vi "Master_IMUMain.vi"(8 "error in":errorcluster, 11 "VISA Refnum out":refnum<visa-resource-name>) -> (0 "error out":errorcluster)   [LabVIEW 2018]
doc: "VI dedicated to reading and processing incoming data from IMU (SBG Ellipse)."
uses:
  TypeDef_LoopPeriods.ctl
  TypeDef_IMUData.ctl
panel:
  out "Data skipped":bool
  out "buffer length":i32
  out "msg_id":string
  # "."
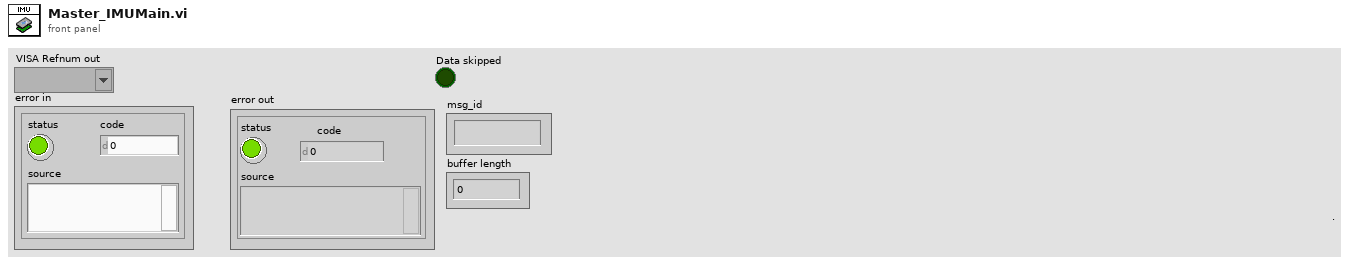
[diagram p1: front panel]
types:
  T1 = typedef "TypeDef_LoopPeriods.ctl" = cluster{"Control Period":i64, "DAQ Period":u32, "IMU Period":u32, "CAN Period":i64, "Nav Period":u32}
  T2 = typedef "TypeDef_IMUData.ctl" = cluster{"x acceleration (g)":dbl, "Pressure (psia)":dbl, "Temperature (F)":dbl}
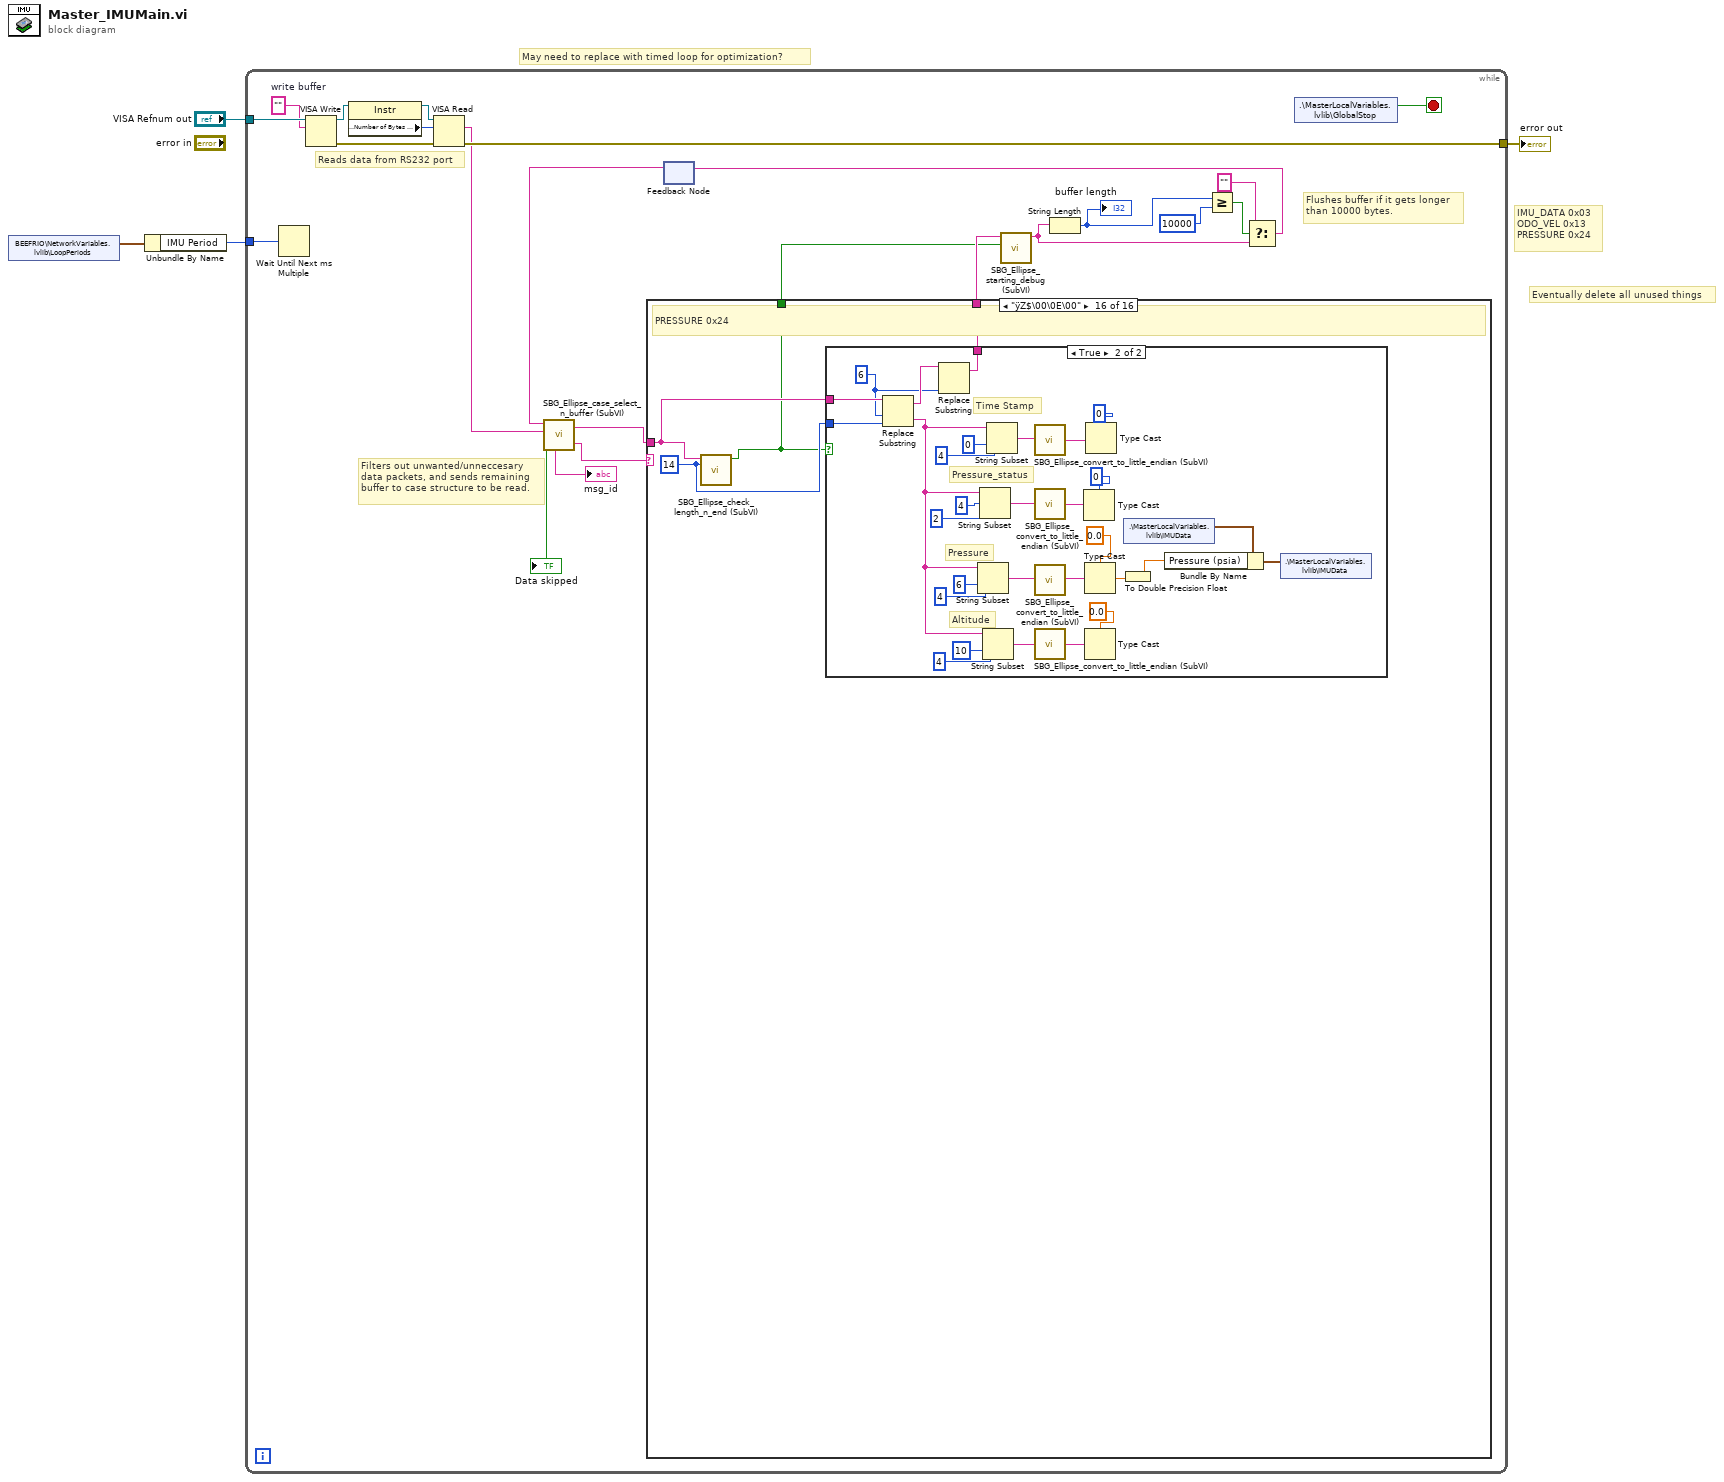
[diagram p0: block diagram]
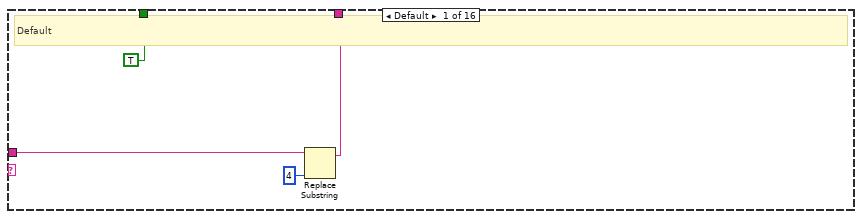
[diagram p2: hidden frame]
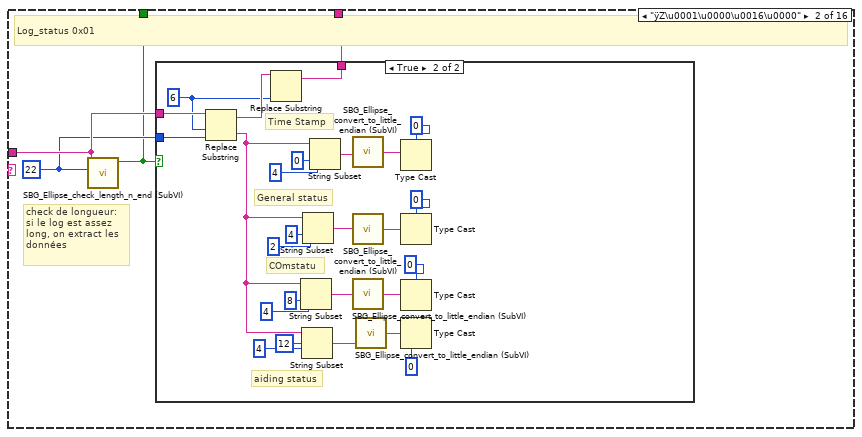
[diagram p3: hidden frame]
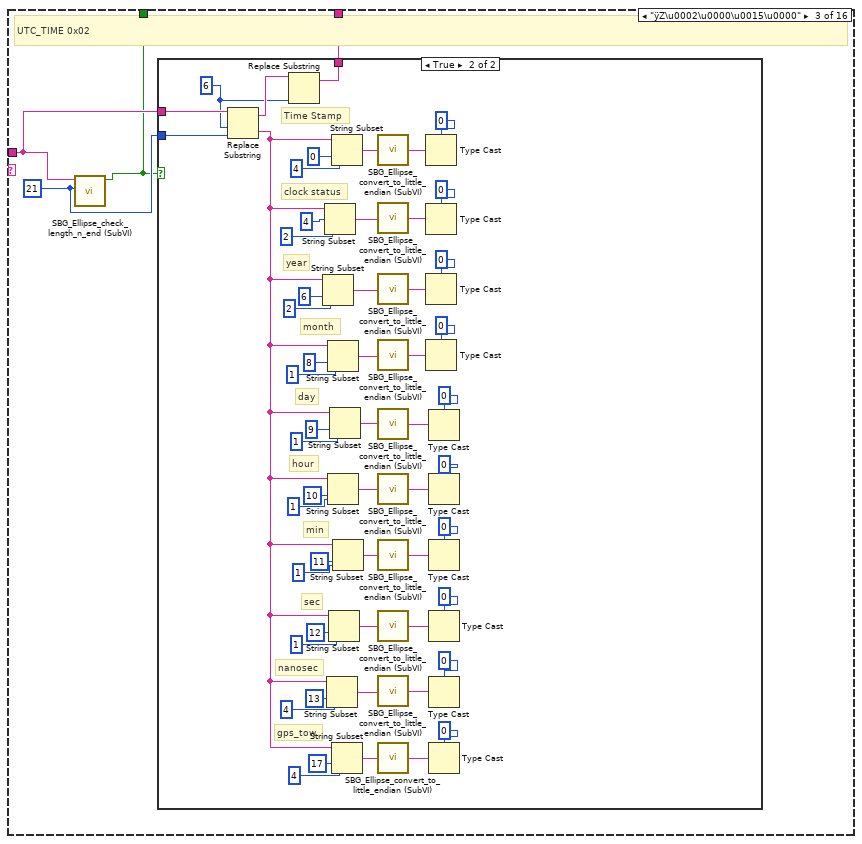
[diagram p5: hidden frame]
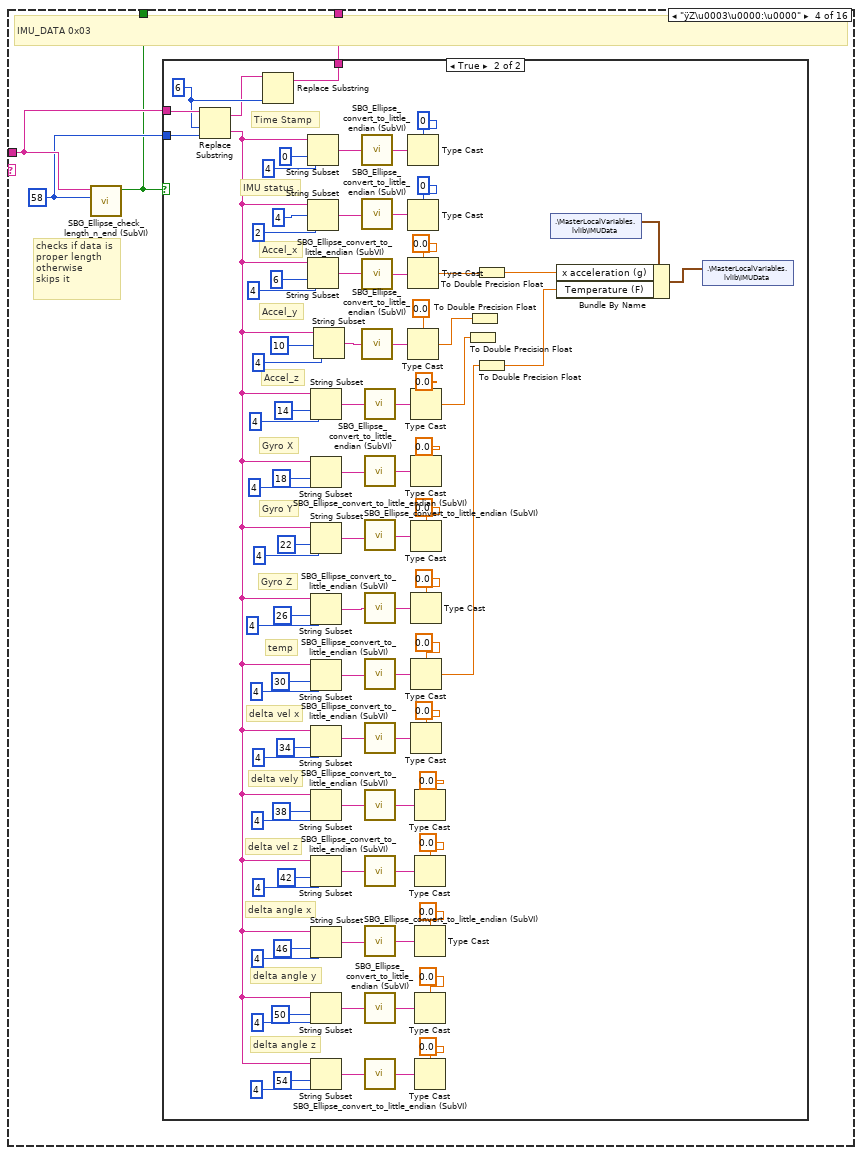
[diagram p7: hidden frame]
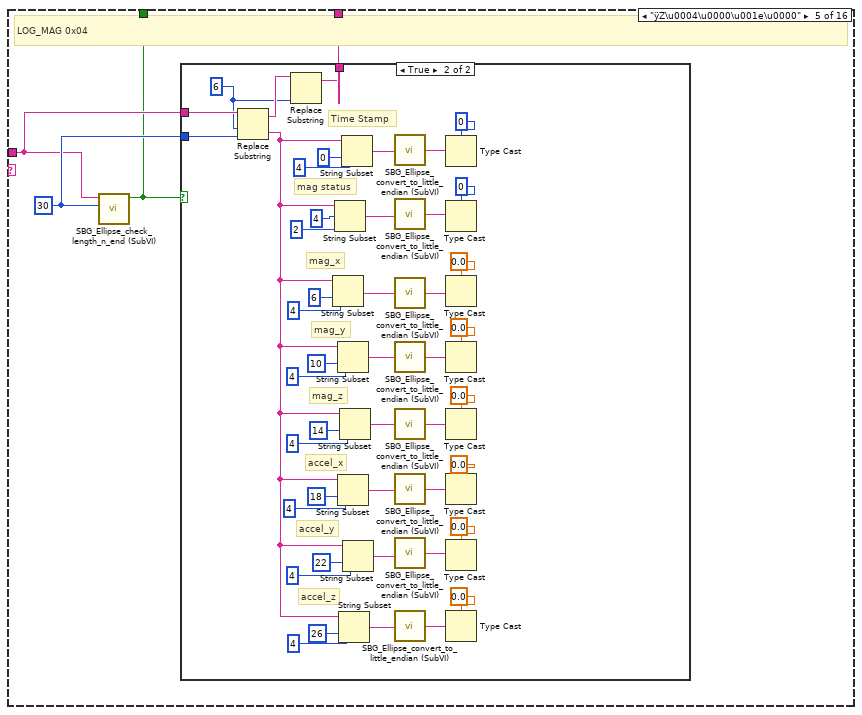
[diagram p9: hidden frame]
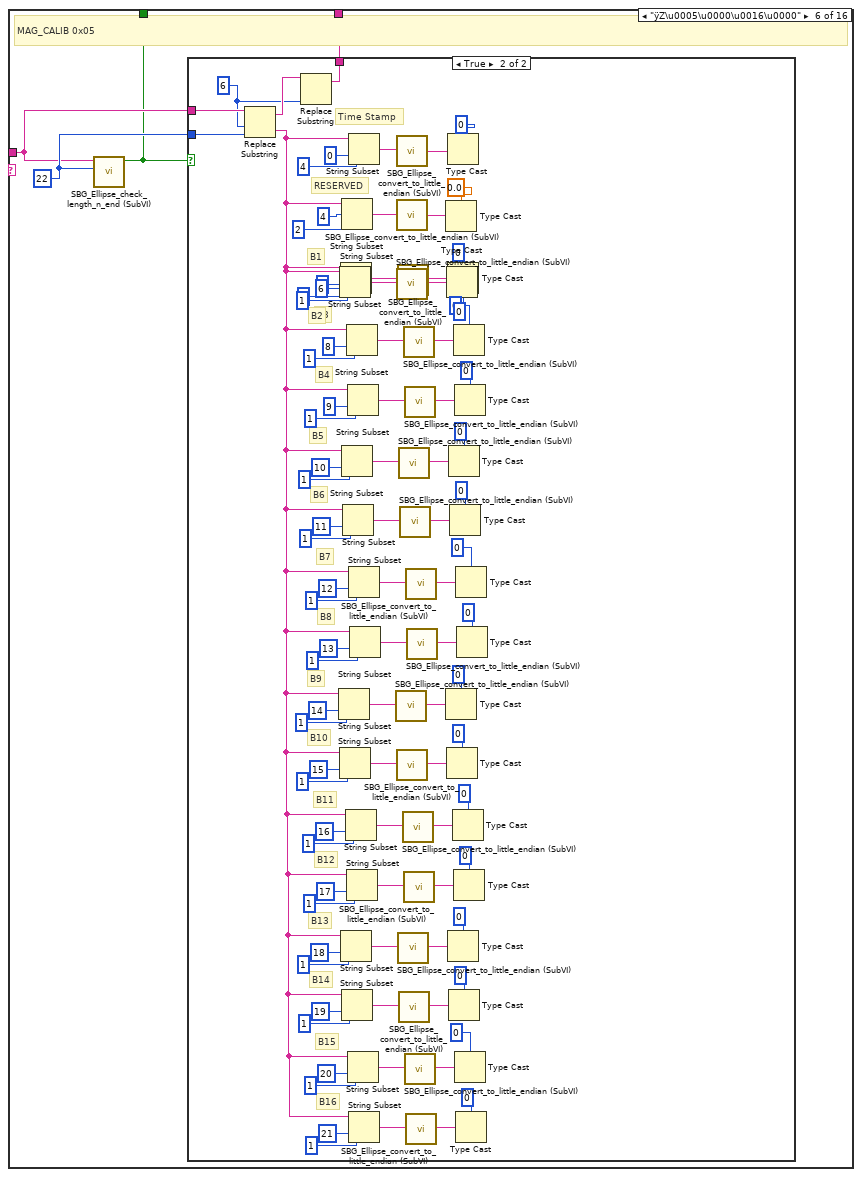
[diagram p11: hidden frame]
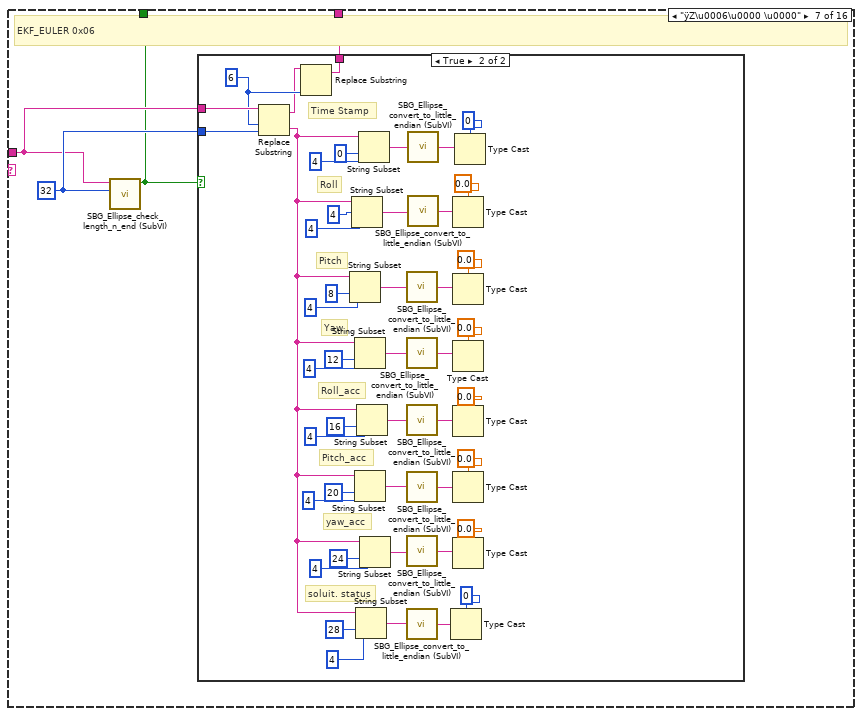
[diagram p13: hidden frame]
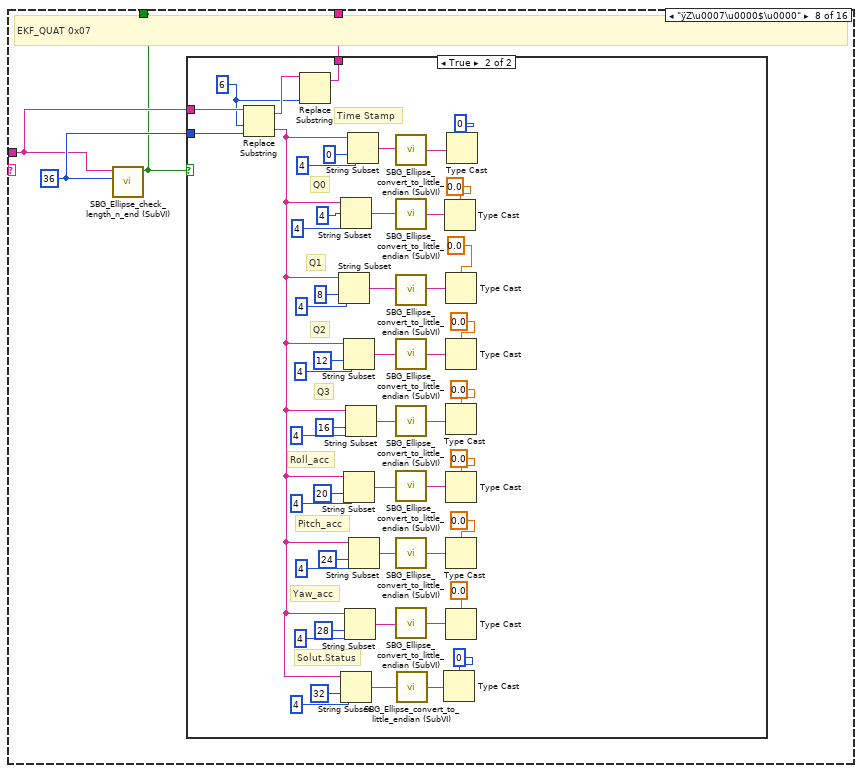
[diagram p15: hidden frame]
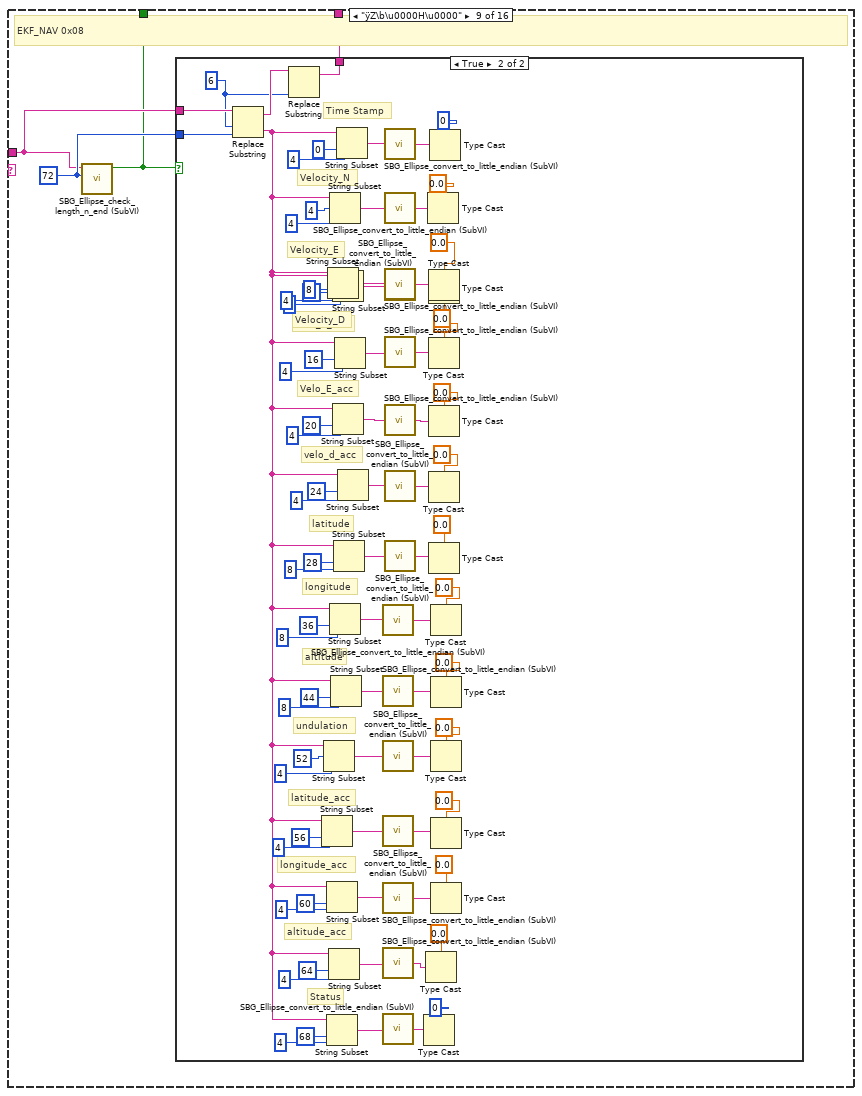
[diagram p17: hidden frame]
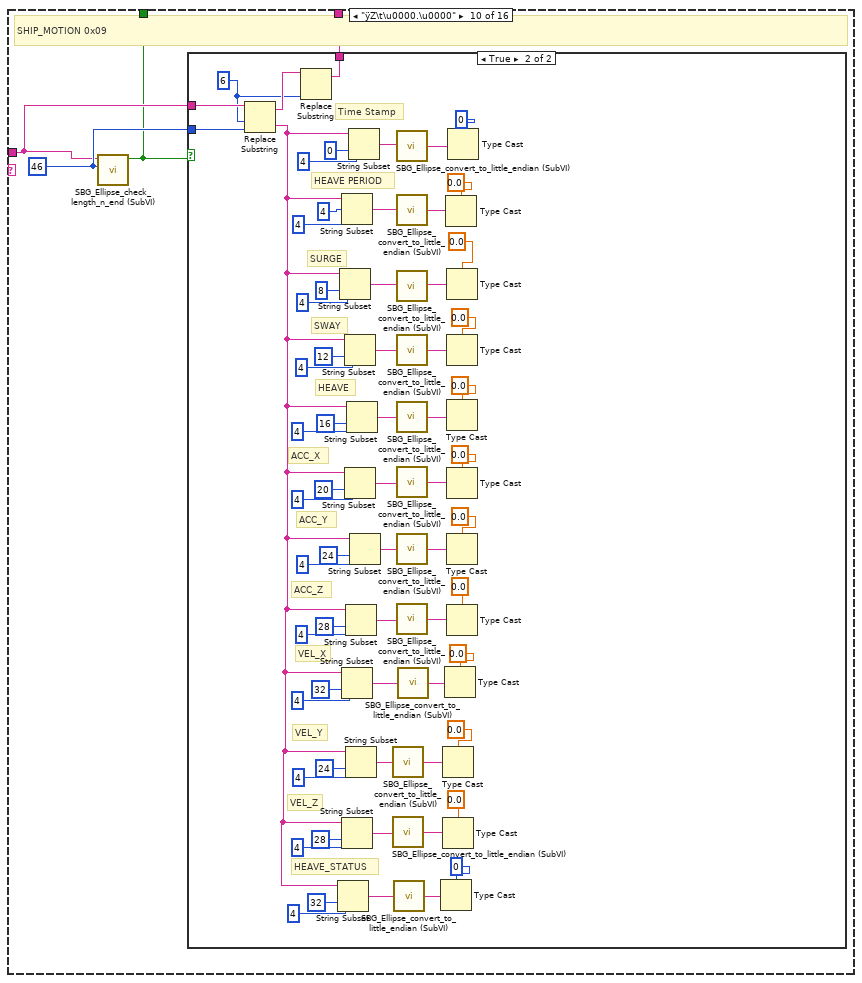
[diagram p19: hidden frame]
diagram:
  # "Eventually delete all unused things"
  # "May need to replace with timed loop for optimization?"
  # "IMU_DATA 0x03\nODO_VEL 0x13\nPRESSURE 0x24"
  n1 = shared-variable "BEEFRIO\\NetworkVariables.lvlib\\LoopPeriods"() -> (w2:T1)  [unwired: 1 in, 1 out]
  n2 = Unbundle By Name(w2) -> ("IMU Period"=w1:u32)
  n3 = while {
    tunnel: "VISA Refnum out" -> [w27]
    tunnel: [w21] -> w3
    tunnel: w1 -> [w11]
    stop <- w10 stop-if-true
    w22 = ""  # write buffer
    # "Filters out unwanted/unneccesary \ndata packets, and sends remaining\nbuffer to case structure to be read."
    # "Reads data from RS232 port"
    # "Flushes buffer if it gets longer\nthan 10000 bytes."
    n4 = Wait Until Next ms Multiple(millisecond multiple=w11) -> ()  [unwired: 1 out]
    n5 = VISA Write(VISA resource name=w27, write buffer=w22) -> (VISA resource name out=w23:refnum<visa-resource-name>, error out=w26:errorcluster)  [unwired: 1 in, 1 out]
    n6 = property class="Instr"(reference=w23) -> (reference out=w24:refnum<visa-resource-name>, "Serial Settings:Number of Bytes at Serial Port"=w25:u32)  [unwired: 1 in, 1 out]
    n7 = VISA Read(VISA resource name=w24, byte count=w25, error in (no error)=w26) -> (read buffer=w19:string, error out=w21:errorcluster)  [unwired: 2 out]
    n8 = feedback #1() -> (w20:string)  [unwired: 1 in]
    n9 = call "SBG_Ellipse_case_select_n_buffer (SubVI).vi"("new data in"=w19, "buffer data in"=w20) -> ("case_selector"=w7:string, "data out"=w8:string, "msg_id"=→"msg_id":string, "Data skipped"=→"Data skipped":bool)  [unwired: 2 in]
    n10 = case shown="\"ÿZ$\\00\\0E\\00\"" w7 {
      tunnel: w8 -> [w30 w34 w66 w126 w220 w271 w371 w423 w479 w565 w634 w702 w778 w824 w851 w892]
      tunnel: [w29 w35 w64 w127 w219 w270 w372 w422 w478 w563 w636 w701 w777 w823 w850 w891] -> w9
      tunnel: [TRUE ("Boolean") w32 w63 w124 w218 w269 w370 w421 w477 w564 w635 w700 w776 w822 w849 w890] -> w6
      frame Default {
        # "Default"
        n11 = Replace Substring(2:4 ("length (len. of substring)"), 5:w30) -> (1:w29:string)  [unwired: 2 in, 1 out]
      }
      frame "ÿZ\u0001\u0000\u0016\u0000" {
        w33 = 22 ("x")
        # "check de longueur:\nsi le log est assez\nlong, on extract les \ndonnées"
        # "Log_status 0x01"
        n12 = call "SBG_Ellipse_check_length_n_end (SubVI).vi"("x"=w33, "input String"=w34) -> ("is data ok?"=w32:bool)  [unwired: 7 in, 2 out]
        n13 = case shown="True" w32 {
          tunnel: w34 -> [w36 w62]
          tunnel: [w36 w45] -> w35
          tunnel: w33 -> [_ w52]
          frame False {
          }
          frame True {
            w46 = 6 ("length (len. of substring)")
            # "aiding status"
            # "COmstatu"
            # "General status"
            # "Time Stamp"
            n14 = Replace Substring(2:w52, 3:w46, 5:w62) -> (0:w61:string, 1:w47:string)  [unwired: 1 in]
            n15 = Replace Substring(2:w46, 5:w47) -> (1:w45:string)  [unwired: 2 in, 1 out]
            n16 = String Subset(string=w61, offset (0)=8 ("length (len. of substring)"), length (rest)=4 ("length (len. of substring)")) -> (substring=w43:string)
            n17 = String Subset(string=w61, offset (0)=12 ("length (len. of substring)"), length (rest)=4 ("length (len. of substring)")) -> (substring=w44:string)
            n18 = String Subset(string=w61, offset (0)=4 ("length (len. of substring)"), length (rest)=2 ("length (len. of substring)")) -> (substring=w42:string)
            n19 = String Subset(string=w61, offset (0)=0 ("length (len. of substring)"), length (rest)=4 ("length (len. of substring)")) -> (substring=w41:string)
            n20 = call "SBG_Ellipse_convert_to_little_endian (SubVI).vi"("string"=w41) -> ("String"=w40:string)  [unwired: 4 in]
            n21 = call "SBG_Ellipse_convert_to_little_endian (SubVI).vi"("string"=w42) -> ("String"=w39:string)  [unwired: 4 in]
            n22 = call "SBG_Ellipse_convert_to_little_endian (SubVI).vi"("string"=w43) -> ("String"=w38:string)  [unwired: 4 in]
            n23 = call "SBG_Ellipse_convert_to_little_endian (SubVI).vi"("string"=w44) -> ("String"=w37:string)  [unwired: 4 in]
            n24 = Type Cast(type=u32 0, x=w40) -> ()  [unwired: 1 out]
            n25 = Type Cast(type=u16 0, x=w39) -> ()  [unwired: 1 out]
            n26 = Type Cast(type=u32 0, x=w38) -> ()  [unwired: 1 out]
            n27 = Type Cast(type=u32 0, x=w37) -> ()  [unwired: 1 out]
          }
        }
      }
      frame "ÿZ\u0002\u0000\u0015\u0000" {
        w65 = 21 ("x")
        # "UTC_TIME 0x02"
        n28 = call "SBG_Ellipse_check_length_n_end (SubVI).vi"("x"=w65, "input String"=w66) -> ("is data ok?"=w63:bool)  [unwired: 7 in, 2 out]
        n29 = case shown="True" w63 {
          tunnel: w66 -> [w67 w123]
          tunnel: [w67 w88] -> w64
          tunnel: w65 -> [_ w101]
          frame False {
          }
          frame True {
            w89 = 6 ("length (len. of substring)")
            # "gps_tow"
            # "nanosec"
            # "sec"
            # "min"
            # "hour"
            # "day"
            # "month"
            # "year"
            # "clock status"
            # "Time Stamp"
            n30 = Replace Substring(2:w101, 3:w89, 5:w123) -> (0:w102:string, 1:w90:string)  [unwired: 1 in]
            n31 = Replace Substring(2:w89, 5:w90) -> (1:w88:string)  [unwired: 2 in, 1 out]
            n32 = String Subset(string=w102, offset (0)=6 ("length (len. of substring)"), length (rest)=2 ("length (len. of substring)")) -> (substring=w83:string)
            n33 = String Subset(string=w102, offset (0)=4 ("length (len. of substring)"), length (rest)=2 ("length (len. of substring)")) -> (substring=w85:string)
            n34 = String Subset(string=w102, offset (0)=13 ("length (len. of substring)"), length (rest)=4 ("length (len. of substring)")) -> (substring=w70:string)
            n35 = String Subset(string=w102, offset (0)=8 ("length (len. of substring)"), length (rest)=1 ("length (len. of substring)")) -> (substring=w81:string)
            n36 = String Subset(string=w102, offset (0)=10 ("length (len. of substring)"), length (rest)=1 ("length (len. of substring)")) -> (substring=w77:string)
            n37 = String Subset(string=w102, offset (0)=12 ("length (len. of substring)"), length (rest)=1 ("length (len. of substring)")) -> (substring=w73:string)
            n38 = String Subset(string=w102, offset (0)=9 ("length (len. of substring)"), length (rest)=1 ("length (len. of substring)")) -> (substring=w79:string)
            n39 = String Subset(string=w102, offset (0)=0 ("length (len. of substring)"), length (rest)=4 ("length (len. of substring)")) -> (substring=w87:string)
            n40 = String Subset(string=w102, offset (0)=17 ("length (len. of substring)"), length (rest)=4 ("length (len. of substring)")) -> (substring=w69:string)
            n41 = String Subset(string=w102, offset (0)=11 ("length (len. of substring)"), length (rest)=1 ("length (len. of substring)")) -> (substring=w75:string)
            n42 = call "SBG_Ellipse_convert_to_little_endian (SubVI).vi"("string"=w87) -> ("String"=w86:string)  [unwired: 4 in]
            n43 = call "SBG_Ellipse_convert_to_little_endian (SubVI).vi"("string"=w85) -> ("String"=w84:string)  [unwired: 4 in]
            n44 = call "SBG_Ellipse_convert_to_little_endian (SubVI).vi"("string"=w83) -> ("String"=w82:string)  [unwired: 4 in]
            n45 = call "SBG_Ellipse_convert_to_little_endian (SubVI).vi"("string"=w81) -> ("String"=w80:string)  [unwired: 4 in]
            n46 = call "SBG_Ellipse_convert_to_little_endian (SubVI).vi"("string"=w79) -> ("String"=w78:string)  [unwired: 4 in]
            n47 = call "SBG_Ellipse_convert_to_little_endian (SubVI).vi"("string"=w77) -> ("String"=w76:string)  [unwired: 4 in]
            n48 = call "SBG_Ellipse_convert_to_little_endian (SubVI).vi"("string"=w75) -> ("String"=w74:string)  [unwired: 4 in]
            n49 = call "SBG_Ellipse_convert_to_little_endian (SubVI).vi"("string"=w73) -> ("String"=w72:string)  [unwired: 4 in]
            n50 = call "SBG_Ellipse_convert_to_little_endian (SubVI).vi"("string"=w70) -> ("String"=w71:string)  [unwired: 4 in]
            n51 = call "SBG_Ellipse_convert_to_little_endian (SubVI).vi"("string"=w69) -> ("String"=w68:string)  [unwired: 4 in]
            n52 = Type Cast(type=u32 0, x=w86) -> ()  [unwired: 1 out]
            n53 = Type Cast(type=u16 0, x=w84) -> ()  [unwired: 1 out]
            n54 = Type Cast(type=u16 0, x=w82) -> ()  [unwired: 1 out]
            n55 = Type Cast(type=u8 0, x=w80) -> ()  [unwired: 1 out]
            n56 = Type Cast(type=u8 0, x=w78) -> ()  [unwired: 1 out]
            n57 = Type Cast(type=u8 0, x=w76) -> ()  [unwired: 1 out]
            n58 = Type Cast(type=u8 0, x=w74) -> ()  [unwired: 1 out]
            n59 = Type Cast(type=u8 0, x=w72) -> ()  [unwired: 1 out]
            n60 = Type Cast(type=u32 0, x=w71) -> ()  [unwired: 1 out]
            n61 = Type Cast(type=u32 0, x=w68) -> ()  [unwired: 1 out]
          }
        }
      }
      frame "ÿZ\u0003\u0000:\u0000" {
        w125 = 58 ("x")
        # "checks if data is\nproper length\notherwise\nskips it"
        # "IMU_DATA 0x03"
        n62 = call "SBG_Ellipse_check_length_n_end (SubVI).vi"("x"=w125, "input String"=w126) -> ("is data ok?"=w124:bool)  [unwired: 7 in, 2 out]
        n63 = case shown="True" w124 {
          tunnel: w126 -> [w128 w217]
          tunnel: [w128 w169] -> w127
          tunnel: w125 -> [_ w196]
          frame False {
          }
          frame True {
            w168 = 6 ("length (len. of substring)")
            # "delta angle z"
            # "delta angle y"
            # "delta angle x"
            # "delta vel z"
            # "delta vely"
            # "delta vel x"
            # "temp"
            # "Gyro Z"
            # "Gyro Y"
            # "Gyro X"
            # "Accel_z"
            # "Accel_y"
            # "Accel_x"
            # "IMU status"
            # "Time Stamp"
            n64 = Replace Substring(2:w196, 3:w168, 5:w217) -> (0:w185:string, 1:w167:string)  [unwired: 1 in]
            n65 = Replace Substring(2:w168, 5:w167) -> (1:w169:string)  [unwired: 2 in, 1 out]
            n66 = String Subset(string=w185, offset (0)=0 ("length (len. of substring)"), length (rest)=4 ("length (len. of substring)")) -> (substring=w140:string)
            n67 = String Subset(string=w185, offset (0)=4 ("length (len. of substring)"), length (rest)=2 ("length (len. of substring)")) -> (substring=w139:string)
            n68 = String Subset(string=w185, offset (0)=6 ("length (len. of substring)"), length (rest)=4 ("length (len. of substring)")) -> (substring=w164:string)
            n69 = String Subset(string=w185, offset (0)=14 ("length (len. of substring)"), length (rest)=4 ("length (len. of substring)")) -> (substring=w165:string)
            n70 = String Subset(string=w185, offset (0)=18 ("length (len. of substring)"), length (rest)=4 ("length (len. of substring)")) -> (substring=w145:string)
            n71 = String Subset(string=w185, offset (0)=22 ("length (len. of substring)"), length (rest)=4 ("length (len. of substring)")) -> (substring=w144:string)
            n72 = String Subset(string=w185, offset (0)=26 ("length (len. of substring)"), length (rest)=4 ("length (len. of substring)")) -> (substring=w143:string)
            n73 = String Subset(string=w185, offset (0)=30 ("length (len. of substring)"), length (rest)=4 ("length (len. of substring)")) -> (substring=w148:string)
            n74 = String Subset(string=w185, offset (0)=34 ("length (len. of substring)"), length (rest)=4 ("length (len. of substring)")) -> (substring=w149:string)
            n75 = String Subset(string=w185, offset (0)=38 ("length (len. of substring)"), length (rest)=4 ("length (len. of substring)")) -> (substring=w160:string)
            n76 = String Subset(string=w185, offset (0)=42 ("length (len. of substring)"), length (rest)=4 ("length (len. of substring)")) -> (substring=w153:string)
            n77 = String Subset(string=w185, offset (0)=46 ("length (len. of substring)"), length (rest)=4 ("length (len. of substring)")) -> (substring=w154:string)
            n78 = String Subset(string=w185, offset (0)=50 ("length (len. of substring)"), length (rest)=4 ("length (len. of substring)")) -> (substring=w159:string)
            n79 = String Subset(string=w185, offset (0)=54 ("length (len. of substring)"), length (rest)=4 ("length (len. of substring)")) -> (substring=w158:string)
            n80 = String Subset(string=w185, offset (0)=10 ("length (len. of substring)"), length (rest)=4 ("length (len. of substring)")) -> (substring=w163:string)
            n81 = call "SBG_Ellipse_convert_to_little_endian (SubVI).vi"("string"=w140) -> ("String"=w137:string)  [unwired: 4 in]
            n82 = call "SBG_Ellipse_convert_to_little_endian (SubVI).vi"("string"=w139) -> ("String"=w138:string)  [unwired: 4 in]
            n83 = call "SBG_Ellipse_convert_to_little_endian (SubVI).vi"("string"=w164) -> ("String"=w161:string)  [unwired: 4 in]
            n84 = call "SBG_Ellipse_convert_to_little_endian (SubVI).vi"("string"=w163) -> ("String"=w162:string)  [unwired: 4 in]
            n85 = call "SBG_Ellipse_convert_to_little_endian (SubVI).vi"("string"=w165) -> ("String"=w166:string)  [unwired: 4 in]
            n86 = call "SBG_Ellipse_convert_to_little_endian (SubVI).vi"("string"=w145) -> ("String"=w146:string)  [unwired: 4 in]
            n87 = call "SBG_Ellipse_convert_to_little_endian (SubVI).vi"("string"=w144) -> ("String"=w141:string)  [unwired: 4 in]
            n88 = call "SBG_Ellipse_convert_to_little_endian (SubVI).vi"("string"=w143) -> ("String"=w142:string)  [unwired: 4 in]
            n89 = call "SBG_Ellipse_convert_to_little_endian (SubVI).vi"("string"=w148) -> ("String"=w147:string)  [unwired: 4 in]
            n90 = call "SBG_Ellipse_convert_to_little_endian (SubVI).vi"("string"=w149) -> ("String"=w150:string)  [unwired: 4 in]
            n91 = call "SBG_Ellipse_convert_to_little_endian (SubVI).vi"("string"=w160) -> ("String"=w151:string)  [unwired: 4 in]
            n92 = call "SBG_Ellipse_convert_to_little_endian (SubVI).vi"("string"=w153) -> ("String"=w152:string)  [unwired: 4 in]
            n93 = call "SBG_Ellipse_convert_to_little_endian (SubVI).vi"("string"=w154) -> ("String"=w155:string)  [unwired: 4 in]
            n94 = call "SBG_Ellipse_convert_to_little_endian (SubVI).vi"("string"=w159) -> ("String"=w156:string)  [unwired: 4 in]
            n95 = call "SBG_Ellipse_convert_to_little_endian (SubVI).vi"("string"=w158) -> ("String"=w157:string)  [unwired: 4 in]
            n96 = Type Cast(type=u32 0, x=w137) -> ()  [unwired: 1 out]
            n97 = Type Cast(type=u16 0, x=w138) -> ()  [unwired: 1 out]
            n98 = Type Cast(type=sgl 0.0, x=w161) -> (*(type *) &x=w136:sgl)
            n99 = Type Cast(type=sgl 0.0, x=w162) -> (*(type *) &x=w130:sgl)
            n100 = Type Cast(type=sgl 0.0, x=w166) -> (*(type *) &x=w129:sgl)
            n101 = Type Cast(type=sgl 0.0, x=w146) -> ()  [unwired: 1 out]
            n102 = Type Cast(type=sgl 0.0, x=w141) -> ()  [unwired: 1 out]
            n103 = Type Cast(type=sgl 0.0, x=w142) -> ()  [unwired: 1 out]
            n104 = Type Cast(type=sgl 0.0, x=w147) -> (*(type *) &x=w135:sgl)
            n105 = Type Cast(type=sgl 0.0, x=w150) -> ()  [unwired: 1 out]
            n106 = Type Cast(type=sgl 0.0, x=w151) -> ()  [unwired: 1 out]
            n107 = Type Cast(type=sgl 0.0, x=w152) -> ()  [unwired: 1 out]
            n108 = Type Cast(type=sgl 0.0, x=w155) -> ()  [unwired: 1 out]
            n109 = Type Cast(type=sgl 0.0, x=w156) -> ()  [unwired: 1 out]
            n110 = Type Cast(type=sgl 0.0, x=w157) -> ()  [unwired: 1 out]
            n111 = To Double Precision Float(number=w129) -> ()  [unwired: 1 out]
            n112 = To Double Precision Float(number=w130) -> ()  [unwired: 1 out]
            n113 = To Double Precision Float(number=w136) -> (double precision float=w132:dbl)
            n114 = To Double Precision Float(number=w135) -> (double precision float=w131:dbl)
            n115 = shared-variable ".\\MasterLocalVariables.lvlib\\IMUData"() -> (w134:T2)  [unwired: 1 in, 1 out]
            n116 = Bundle By Name(cluster=w134, "x acceleration (g)"=w132, "Temperature (F)"=w131) -> (w133:T2)
            n117 = shared-variable ".\\MasterLocalVariables.lvlib\\IMUData"(w133) -> ()  [unwired: 1 in, 1 out]
          }
        }
      }
      frame "ÿZ\u0004\u0000\u001e\u0000" {
        w221 = 30 ("x")
        # "LOG_MAG 0x04"
        n118 = call "SBG_Ellipse_check_length_n_end (SubVI).vi"("x"=w221, "input String"=w220) -> ("is data ok?"=w218:bool)  [unwired: 7 in, 2 out]
        n119 = case shown="True" w218 {
          tunnel: w220 -> [w222 w268]
          tunnel: [w222 w239] -> w219
          tunnel: w221 -> [_ w250]
          frame False {
          }
          frame True {
            w240 = 6 ("length (len. of substring)")
            # "accel_z"
            # "accel_y"
            # "accel_x"
            # "mag_z"
            # "mag_y"
            # "mag_x"
            # "mag status"
            # "Time Stamp"
            n120 = Replace Substring(2:w250, 3:w240, 5:w268) -> (0:w251:string, 1:w241:string)  [unwired: 1 in]
            n121 = Replace Substring(2:w240, 5:w241) -> (1:w239:string)  [unwired: 2 in, 1 out]
            n122 = String Subset(string=w251, offset (0)=6 ("length (len. of substring)"), length (rest)=4 ("length (len. of substring)")) -> (substring=w234:string)
            n123 = String Subset(string=w251, offset (0)=4 ("length (len. of substring)"), length (rest)=2 ("length (len. of substring)")) -> (substring=w236:string)
            n124 = String Subset(string=w251, offset (0)=10 ("length (len. of substring)"), length (rest)=4 ("length (len. of substring)")) -> (substring=w231:string)
            n125 = String Subset(string=w251, offset (0)=18 ("length (len. of substring)"), length (rest)=4 ("length (len. of substring)")) -> (substring=w228:string)
            n126 = String Subset(string=w251, offset (0)=26 ("length (len. of substring)"), length (rest)=4 ("length (len. of substring)")) -> (substring=w226:string)
            n127 = String Subset(string=w251, offset (0)=14 ("length (len. of substring)"), length (rest)=4 ("length (len. of substring)")) -> (substring=w230:string)
            n128 = String Subset(string=w251, offset (0)=0 ("length (len. of substring)"), length (rest)=4 ("length (len. of substring)")) -> (substring=w238:string)
            n129 = String Subset(string=w251, offset (0)=22 ("length (len. of substring)"), length (rest)=4 ("length (len. of substring)")) -> (substring=w227:string)
            n130 = call "SBG_Ellipse_convert_to_little_endian (SubVI).vi"("string"=w238) -> ("String"=w237:string)  [unwired: 4 in]
            n131 = call "SBG_Ellipse_convert_to_little_endian (SubVI).vi"("string"=w236) -> ("String"=w235:string)  [unwired: 4 in]
            n132 = call "SBG_Ellipse_convert_to_little_endian (SubVI).vi"("string"=w234) -> ("String"=w233:string)  [unwired: 4 in]
            n133 = call "SBG_Ellipse_convert_to_little_endian (SubVI).vi"("string"=w231) -> ("String"=w232:string)  [unwired: 4 in]
            n134 = call "SBG_Ellipse_convert_to_little_endian (SubVI).vi"("string"=w230) -> ("String"=w229:string)  [unwired: 4 in]
            n135 = call "SBG_Ellipse_convert_to_little_endian (SubVI).vi"("string"=w228) -> ("String"=w223:string)  [unwired: 4 in]
            n136 = call "SBG_Ellipse_convert_to_little_endian (SubVI).vi"("string"=w227) -> ("String"=w224:string)  [unwired: 4 in]
            n137 = call "SBG_Ellipse_convert_to_little_endian (SubVI).vi"("string"=w226) -> ("String"=w225:string)  [unwired: 4 in]
            n138 = Type Cast(type=u32 0, x=w237) -> ()  [unwired: 1 out]
            n139 = Type Cast(type=u16 0, x=w235) -> ()  [unwired: 1 out]
            n140 = Type Cast(type=sgl 0.0, x=w233) -> ()  [unwired: 1 out]
            n141 = Type Cast(type=sgl 0.0, x=w232) -> ()  [unwired: 1 out]
            n142 = Type Cast(type=sgl 0.0, x=w229) -> ()  [unwired: 1 out]
            n143 = Type Cast(type=sgl 0.0, x=w223) -> ()  [unwired: 1 out]
            n144 = Type Cast(type=sgl 0.0, x=w224) -> ()  [unwired: 1 out]
            n145 = Type Cast(type=sgl 0.0, x=w225) -> ()  [unwired: 1 out]
          }
        }
      }
      frame "ÿZ\u0005\u0000\u0016\u0000" {
        w272 = 22 ("x")
        # "MAG_CALIB 0x05"
        n146 = call "SBG_Ellipse_check_length_n_end (SubVI).vi"("x"=w272, "input String"=w271) -> ("is data ok?"=w269:bool)  [unwired: 7 in, 2 out]
        n147 = case shown="True" w269 {
          tunnel: w271 -> [w273 w369]
          tunnel: [w273 w356] -> w270
          tunnel: w272 -> [_ w362]
          frame False {
          }
          frame True {
            w357 = 6 ("length (len. of substring)")
            # "B16"
            # "B15"
            # "B14"
            # "B13"
            # "B12"
            # "B11"
            # "B10"
            # "B9"
            # "B8"
            # "B7"
            # "B6"
            # "B5"
            # "B4"
            # "B3"
            # "B2"
            # "B1"
            # "RESERVED"
            # "Time Stamp"
            n148 = Replace Substring(2:w362, 3:w357, 5:w369) -> (0:w274:string, 1:w358:string)  [unwired: 1 in]
            n149 = Replace Substring(2:w357, 5:w358) -> (1:w356:string)  [unwired: 2 in, 1 out]
            n150 = String Subset(string=w274, offset (0)=14 ("length (len. of substring)"), length (rest)=1 ("length (len. of substring)")) -> (substring=w278:string)
            n151 = String Subset(string=w274, offset (0)=6 ("length (len. of substring)"), length (rest)=1 ("length (len. of substring)")) -> (substring=w351:string)
            n152 = String Subset(string=w274, offset (0)=15 ("length (len. of substring)"), length (rest)=1 ("length (len. of substring)")) -> (substring=w281:string)
            n153 = String Subset(string=w274, offset (0)=7 ("length (len. of substring)"), length (rest)=1 ("length (len. of substring)")) -> (substring=w348:string)
            n154 = String Subset(string=w274, offset (0)=18 ("length (len. of substring)"), length (rest)=1 ("length (len. of substring)")) -> (substring=w311:string)
            n155 = String Subset(string=w274, offset (0)=4 ("length (len. of substring)"), length (rest)=2 ("length (len. of substring)")) -> (substring=w353:string)
            n156 = String Subset(string=w274, offset (0)=10 ("length (len. of substring)"), length (rest)=1 ("length (len. of substring)")) -> (substring=w318:string)
            n157 = String Subset(string=w274, offset (0)=19 ("length (len. of substring)"), length (rest)=1 ("length (len. of substring)")) -> (substring=w308:string)
            n158 = String Subset(string=w274, offset (0)=11 ("length (len. of substring)"), length (rest)=1 ("length (len. of substring)")) -> (substring=w321:string)
            n159 = String Subset(string=w274, offset (0)=16 ("length (len. of substring)"), length (rest)=1 ("length (len. of substring)")) -> (substring=w289:string)
            n160 = String Subset(string=w274, offset (0)=8 ("length (len. of substring)"), length (rest)=1 ("length (len. of substring)")) -> (substring=w340:string)
            n161 = String Subset(string=w274, offset (0)=17 ("length (len. of substring)"), length (rest)=1 ("length (len. of substring)")) -> (substring=w286:string)
            n162 = String Subset(string=w274, offset (0)=9 ("length (len. of substring)"), length (rest)=1 ("length (len. of substring)")) -> (substring=w343:string)
            n163 = String Subset(string=w274, offset (0)=20 ("length (len. of substring)"), length (rest)=1 ("length (len. of substring)")) -> (substring=w300:string)
            n164 = String Subset(string=w274, offset (0)=0 ("length (len. of substring)"), length (rest)=4 ("length (len. of substring)")) -> (substring=w355:string)
            n165 = String Subset(string=w274, offset (0)=12 ("length (len. of substring)"), length (rest)=1 ("length (len. of substring)")) -> (substring=w329:string)
            n166 = String Subset(string=w274, offset (0)=21 ("length (len. of substring)"), length (rest)=1 ("length (len. of substring)")) -> (substring=w303:string)
            n167 = String Subset(string=w274, offset (0)=13 ("length (len. of substring)"), length (rest)=1 ("length (len. of substring)")) -> (substring=w326:string)
            n168 = call "SBG_Ellipse_convert_to_little_endian (SubVI).vi"("string"=w278) -> ("String"=w279:string)  [unwired: 4 in]
            n169 = call "SBG_Ellipse_convert_to_little_endian (SubVI).vi"("string"=w355) -> ("String"=w354:string)  [unwired: 4 in]
            n170 = call "SBG_Ellipse_convert_to_little_endian (SubVI).vi"("string"=w353) -> ("String"=w352:string)  [unwired: 4 in]
            n171 = call "SBG_Ellipse_convert_to_little_endian (SubVI).vi"("string"=w351) -> ("String"=w350:string)  [unwired: 4 in]
            n172 = call "SBG_Ellipse_convert_to_little_endian (SubVI).vi"("string"=w281) -> ("String"=w280:string)  [unwired: 4 in]
            n173 = call "SBG_Ellipse_convert_to_little_endian (SubVI).vi"("string"=w348) -> ("String"=w349:string)  [unwired: 4 in]
            n174 = call "SBG_Ellipse_convert_to_little_endian (SubVI).vi"("string"=w311) -> ("String"=w310:string)  [unwired: 4 in]
            n175 = call "SBG_Ellipse_convert_to_little_endian (SubVI).vi"("string"=w318) -> ("String"=w319:string)  [unwired: 4 in]
            n176 = call "SBG_Ellipse_convert_to_little_endian (SubVI).vi"("string"=w308) -> ("String"=w309:string)  [unwired: 4 in]
            n177 = call "SBG_Ellipse_convert_to_little_endian (SubVI).vi"("string"=w321) -> ("String"=w320:string)  [unwired: 4 in]
            n178 = call "SBG_Ellipse_convert_to_little_endian (SubVI).vi"("string"=w289) -> ("String"=w288:string)  [unwired: 4 in]
            n179 = call "SBG_Ellipse_convert_to_little_endian (SubVI).vi"("string"=w340) -> ("String"=w341:string)  [unwired: 4 in]
            n180 = call "SBG_Ellipse_convert_to_little_endian (SubVI).vi"("string"=w286) -> ("String"=w287:string)  [unwired: 4 in]
            n181 = call "SBG_Ellipse_convert_to_little_endian (SubVI).vi"("string"=w343) -> ("String"=w342:string)  [unwired: 4 in]
            n182 = call "SBG_Ellipse_convert_to_little_endian (SubVI).vi"("string"=w300) -> ("String"=w301:string)  [unwired: 4 in]
            n183 = call "SBG_Ellipse_convert_to_little_endian (SubVI).vi"("string"=w329) -> ("String"=w328:string)  [unwired: 4 in]
            n184 = call "SBG_Ellipse_convert_to_little_endian (SubVI).vi"("string"=w303) -> ("String"=w302:string)  [unwired: 4 in]
            n185 = call "SBG_Ellipse_convert_to_little_endian (SubVI).vi"("string"=w326) -> ("String"=w327:string)  [unwired: 4 in]
            n186 = Type Cast(type=sgl 0.0, x=w352) -> ()  [unwired: 1 out]
            n187 = Type Cast(type=u8 0, x=w279) -> ()  [unwired: 1 out]
            n188 = Type Cast(type=u8 0, x=w350) -> ()  [unwired: 1 out]
            n189 = Type Cast(type=u8 0, x=w280) -> ()  [unwired: 1 out]
            n190 = Type Cast(type=u32 0, x=w354) -> ()  [unwired: 1 out]
            n191 = Type Cast(type=u8 0, x=w349) -> ()  [unwired: 1 out]
            n192 = Type Cast(type=u8 0, x=w310) -> ()  [unwired: 1 out]
            n193 = Type Cast(type=u8 0, x=w319) -> ()  [unwired: 1 out]
            n194 = Type Cast(type=u8 0, x=w309) -> ()  [unwired: 1 out]
            n195 = Type Cast(type=u8 0, x=w320) -> ()  [unwired: 1 out]
            n196 = Type Cast(type=u8 0, x=w288) -> ()  [unwired: 1 out]
            n197 = Type Cast(type=u8 0, x=w341) -> ()  [unwired: 1 out]
            n198 = Type Cast(type=u8 0, x=w287) -> ()  [unwired: 1 out]
            n199 = Type Cast(type=u8 0, x=w342) -> ()  [unwired: 1 out]
            n200 = Type Cast(type=u8 0, x=w301) -> ()  [unwired: 1 out]
            n201 = Type Cast(type=u8 0, x=w328) -> ()  [unwired: 1 out]
            n202 = Type Cast(type=u8 0, x=w302) -> ()  [unwired: 1 out]
            n203 = Type Cast(type=u8 0, x=w327) -> ()  [unwired: 1 out]
          }
        }
      }
      frame "ÿZ\u0006\u0000 \u0000" {
        w373 = 32 ("x")
        # "EKF_EULER 0x06"
        n204 = call "SBG_Ellipse_check_length_n_end (SubVI).vi"("x"=w373, "input String"=w371) -> ("is data ok?"=w370:bool)  [unwired: 7 in, 2 out]
        n205 = case shown="True" w370 {
          tunnel: w371 -> [w374 w420]
          tunnel: [w374 w392] -> w372
          tunnel: w373 -> [_ w402]
          frame False {
          }
          frame True {
            w393 = 6 ("length (len. of substring)")
            # "soluit. status"
            # "yaw_acc"
            # "Pitch_acc"
            # "Roll_acc"
            # "Yaw"
            # "Pitch"
            # "Roll"
            # "Time Stamp"
            n206 = Replace Substring(2:w402, 3:w393, 5:w420) -> (0:w403:string, 1:w391:string)  [unwired: 1 in]
            n207 = Replace Substring(2:w393, 5:w391) -> (1:w392:string)  [unwired: 2 in, 1 out]
            n208 = String Subset(string=w403, offset (0)=8 ("length (len. of substring)"), length (rest)=4 ("length (len. of substring)")) -> (substring=w386:string)
            n209 = String Subset(string=w403, offset (0)=4 ("length (len. of substring)"), length (rest)=4 ("length (len. of substring)")) -> (substring=w388:string)
            n210 = String Subset(string=w403, offset (0)=12 ("length (len. of substring)"), length (rest)=4 ("length (len. of substring)")) -> (substring=w384:string)
            n211 = String Subset(string=w403, offset (0)=20 ("length (len. of substring)"), length (rest)=4 ("length (len. of substring)")) -> (substring=w380:string)
            n212 = String Subset(string=w403, offset (0)=28 ("length (len. of substring)"), length (rest)=4 ("length (len. of substring)")) -> (substring=w376:string)
            n213 = String Subset(string=w403, offset (0)=16 ("length (len. of substring)"), length (rest)=4 ("length (len. of substring)")) -> (substring=w382:string)
            n214 = String Subset(string=w403, offset (0)=0 ("length (len. of substring)"), length (rest)=4 ("length (len. of substring)")) -> (substring=w390:string)
            n215 = String Subset(string=w403, offset (0)=24 ("length (len. of substring)"), length (rest)=4 ("length (len. of substring)")) -> (substring=w378:string)
            n216 = call "SBG_Ellipse_convert_to_little_endian (SubVI).vi"("string"=w386) -> ("String"=w385:string)  [unwired: 4 in]
            n217 = call "SBG_Ellipse_convert_to_little_endian (SubVI).vi"("string"=w384) -> ("String"=w383:string)  [unwired: 4 in]
            n218 = call "SBG_Ellipse_convert_to_little_endian (SubVI).vi"("string"=w382) -> ("String"=w381:string)  [unwired: 4 in]
            n219 = call "SBG_Ellipse_convert_to_little_endian (SubVI).vi"("string"=w380) -> ("String"=w379:string)  [unwired: 4 in]
            n220 = call "SBG_Ellipse_convert_to_little_endian (SubVI).vi"("string"=w378) -> ("String"=w377:string)  [unwired: 4 in]
            n221 = call "SBG_Ellipse_convert_to_little_endian (SubVI).vi"("string"=w376) -> ("String"=w375:string)  [unwired: 4 in]
            n222 = call "SBG_Ellipse_convert_to_little_endian (SubVI).vi"("string"=w390) -> ("String"=w389:string)  [unwired: 4 in]
            n223 = call "SBG_Ellipse_convert_to_little_endian (SubVI).vi"("string"=w388) -> ("String"=w387:string)  [unwired: 4 in]
            n224 = Type Cast(type=u32 0, x=w375) -> ()  [unwired: 1 out]
            n225 = Type Cast(type=sgl 0.0, x=w387) -> ()  [unwired: 1 out]
            n226 = Type Cast(type=sgl 0.0, x=w385) -> ()  [unwired: 1 out]
            n227 = Type Cast(type=sgl 0.0, x=w383) -> ()  [unwired: 1 out]
            n228 = Type Cast(type=sgl 0.0, x=w381) -> ()  [unwired: 1 out]
            n229 = Type Cast(type=sgl 0.0, x=w379) -> ()  [unwired: 1 out]
            n230 = Type Cast(type=sgl 0.0, x=w377) -> ()  [unwired: 1 out]
            n231 = Type Cast(type=u32 0, x=w389) -> ()  [unwired: 1 out]
          }
        }
      }
      frame "ÿZ\u0007\u0000$\u0000" {
        w424 = 36 ("x")
        # "EKF_QUAT 0x07"
        n232 = call "SBG_Ellipse_check_length_n_end (SubVI).vi"("x"=w424, "input String"=w423) -> ("is data ok?"=w421:bool)  [unwired: 7 in, 2 out]
        n233 = case shown="True" w421 {
          tunnel: w423 -> [w425 w476]
          tunnel: [w425 w444] -> w422
          tunnel: w424 -> [_ w459]
          frame False {
          }
          frame True {
            w445 = 6 ("length (len. of substring)")
            # "Solut.Status"
            # "Yaw_acc"
            # "Pitch_acc"
            # "Roll_acc"
            # "Q3"
            # "Q2"
            # "Q1"
            # "Q0"
            # "Time Stamp"
            n234 = Replace Substring(2:w459, 3:w445, 5:w476) -> (0:w456:string, 1:w446:string)  [unwired: 1 in]
            n235 = Replace Substring(2:w445, 5:w446) -> (1:w444:string)  [unwired: 2 in, 1 out]
            n236 = String Subset(string=w456, offset (0)=8 ("length (len. of substring)"), length (rest)=4 ("length (len. of substring)")) -> (substring=w439:string)
            n237 = String Subset(string=w456, offset (0)=4 ("length (len. of substring)"), length (rest)=4 ("length (len. of substring)")) -> (substring=w441:string)
            n238 = String Subset(string=w456, offset (0)=32 ("length (len. of substring)"), length (rest)=4 ("length (len. of substring)")) -> (substring=w426:string)
            n239 = String Subset(string=w456, offset (0)=12 ("length (len. of substring)"), length (rest)=4 ("length (len. of substring)")) -> (substring=w437:string)
            n240 = String Subset(string=w456, offset (0)=20 ("length (len. of substring)"), length (rest)=4 ("length (len. of substring)")) -> (substring=w433:string)
            n241 = String Subset(string=w456, offset (0)=28 ("length (len. of substring)"), length (rest)=4 ("length (len. of substring)")) -> (substring=w429:string)
            n242 = String Subset(string=w456, offset (0)=16 ("length (len. of substring)"), length (rest)=4 ("length (len. of substring)")) -> (substring=w435:string)
            n243 = String Subset(string=w456, offset (0)=0 ("length (len. of substring)"), length (rest)=4 ("length (len. of substring)")) -> (substring=w443:string)
            n244 = String Subset(string=w456, offset (0)=24 ("length (len. of substring)"), length (rest)=4 ("length (len. of substring)")) -> (substring=w431:string)
            n245 = call "SBG_Ellipse_convert_to_little_endian (SubVI).vi"("string"=w443) -> ("String"=w442:string)  [unwired: 4 in]
            n246 = call "SBG_Ellipse_convert_to_little_endian (SubVI).vi"("string"=w441) -> ("String"=w440:string)  [unwired: 4 in]
            n247 = call "SBG_Ellipse_convert_to_little_endian (SubVI).vi"("string"=w439) -> ("String"=w438:string)  [unwired: 4 in]
            n248 = call "SBG_Ellipse_convert_to_little_endian (SubVI).vi"("string"=w437) -> ("String"=w436:string)  [unwired: 4 in]
            n249 = call "SBG_Ellipse_convert_to_little_endian (SubVI).vi"("string"=w435) -> ("String"=w434:string)  [unwired: 4 in]
            n250 = call "SBG_Ellipse_convert_to_little_endian (SubVI).vi"("string"=w433) -> ("String"=w432:string)  [unwired: 4 in]
            n251 = call "SBG_Ellipse_convert_to_little_endian (SubVI).vi"("string"=w431) -> ("String"=w430:string)  [unwired: 4 in]
            n252 = call "SBG_Ellipse_convert_to_little_endian (SubVI).vi"("string"=w429) -> ("String"=w428:string)  [unwired: 4 in]
            n253 = call "SBG_Ellipse_convert_to_little_endian (SubVI).vi"("string"=w426) -> ("String"=w427:string)  [unwired: 4 in]
            n254 = Type Cast(type=u32 0, x=w427) -> ()  [unwired: 1 out]
            n255 = Type Cast(type=sgl 0.0, x=w440) -> ()  [unwired: 1 out]
            n256 = Type Cast(type=sgl 0.0, x=w438) -> ()  [unwired: 1 out]
            n257 = Type Cast(type=sgl 0.0, x=w436) -> ()  [unwired: 1 out]
            n258 = Type Cast(type=sgl 0.0, x=w434) -> ()  [unwired: 1 out]
            n259 = Type Cast(type=sgl 0.0, x=w432) -> ()  [unwired: 1 out]
            n260 = Type Cast(type=sgl 0.0, x=w430) -> ()  [unwired: 1 out]
            n261 = Type Cast(type=sgl 0.0, x=w428) -> ()  [unwired: 1 out]
            n262 = Type Cast(type=u32 0, x=w442) -> ()  [unwired: 1 out]
          }
        }
      }
      frame "ÿZ\b\u0000H\u0000" {
        w480 = 72 ("x")
        # "EKF_NAV 0x08"
        n263 = call "SBG_Ellipse_check_length_n_end (SubVI).vi"("x"=w480, "input String"=w479) -> ("is data ok?"=w477:bool)  [unwired: 7 in, 2 out]
        n264 = case shown="True" w477 {
          tunnel: w479 -> [w481 w562]
          tunnel: [w481 w512] -> w478
          tunnel: w480 -> [_ w545]
          frame False {
          }
          frame True {
            w513 = 6 ("length (len. of substring)")
            # "Status"
            # "altitude_acc"
            # "longitude_acc"
            # "latitude_acc"
            # "undulation"
            # "altitude"
            # "longitude"
            # "latitude"
            # "velo_d_acc"
            # "Velo_E_acc"
            # "Velo_n_acc"
            # "Velocity_D"
            # "Velocity_E"
            # "Velocity_N"
            # "Time Stamp"
            n265 = Replace Substring(2:w545, 3:w513, 5:w562) -> (0:w530:string, 1:w514:string)  [unwired: 1 in]
            n266 = Replace Substring(2:w513, 5:w514) -> (1:w512:string)  [unwired: 2 in, 1 out]
            n267 = String Subset(string=w530, offset (0)=56 ("length (len. of substring)"), length (rest)=4 ("length (len. of substring)")) -> (substring=w489:string)
            n268 = String Subset(string=w530, offset (0)=52 ("length (len. of substring)"), length (rest)=4 ("length (len. of substring)")) -> (substring=w491:string)
            n269 = String Subset(string=w530, offset (0)=60 ("length (len. of substring)"), length (rest)=4 ("length (len. of substring)")) -> (substring=w487:string)
            n270 = String Subset(string=w530, offset (0)=68 ("length (len. of substring)"), length (rest)=4 ("length (len. of substring)")) -> (substring=w483:string)
            n271 = String Subset(string=w530, offset (0)=8 ("length (len. of substring)"), length (rest)=4 ("length (len. of substring)")) -> (substring=w507:string)
            n272 = String Subset(string=w530, offset (0)=64 ("length (len. of substring)"), length (rest)=4 ("length (len. of substring)")) -> (substring=w485:string)
            n273 = String Subset(string=w530, offset (0)=4 ("length (len. of substring)"), length (rest)=4 ("length (len. of substring)")) -> (substring=w509:string)
            n274 = String Subset(string=w530, offset (0)=36 ("length (len. of substring)"), length (rest)=8 ("length (len. of substring)")) -> (substring=w495:string)
            n275 = String Subset(string=w530, offset (0)=44 ("length (len. of substring)"), length (rest)=8 ("length (len. of substring)")) -> (substring=w493:string)
            n276 = String Subset(string=w530, offset (0)=12 ("length (len. of substring)"), length (rest)=4 ("length (len. of substring)")) -> (substring=w505:string)
            n277 = String Subset(string=w530, offset (0)=20 ("length (len. of substring)"), length (rest)=4 ("length (len. of substring)")) -> (substring=w501:string)
            n278 = String Subset(string=w530, offset (0)=28 ("length (len. of substring)"), length (rest)=8 ("length (len. of substring)")) -> (substring=w497:string)
            n279 = String Subset(string=w530, offset (0)=16 ("length (len. of substring)"), length (rest)=4 ("length (len. of substring)")) -> (substring=w503:string)
            n280 = String Subset(string=w530, offset (0)=0 ("length (len. of substring)"), length (rest)=4 ("length (len. of substring)")) -> (substring=w511:string)
            n281 = String Subset(string=w530, offset (0)=24 ("length (len. of substring)"), length (rest)=4 ("length (len. of substring)")) -> (substring=w499:string)
            n282 = call "SBG_Ellipse_convert_to_little_endian (SubVI).vi"("string"=w495) -> ("String"=w494:string)  [unwired: 4 in]
            n283 = call "SBG_Ellipse_convert_to_little_endian (SubVI).vi"("string"=w493) -> ("String"=w492:string)  [unwired: 4 in]
            n284 = call "SBG_Ellipse_convert_to_little_endian (SubVI).vi"("string"=w491) -> ("String"=w490:string)  [unwired: 4 in]
            n285 = call "SBG_Ellipse_convert_to_little_endian (SubVI).vi"("string"=w489) -> ("String"=w488:string)  [unwired: 4 in]
            n286 = call "SBG_Ellipse_convert_to_little_endian (SubVI).vi"("string"=w487) -> ("String"=w486:string)  [unwired: 4 in]
            n287 = call "SBG_Ellipse_convert_to_little_endian (SubVI).vi"("string"=w485) -> ("String"=w484:string)  [unwired: 4 in]
            n288 = call "SBG_Ellipse_convert_to_little_endian (SubVI).vi"("string"=w483) -> ("String"=w482:string)  [unwired: 4 in]
            n289 = call "SBG_Ellipse_convert_to_little_endian (SubVI).vi"("string"=w511) -> ("String"=w510:string)  [unwired: 4 in]
            n290 = call "SBG_Ellipse_convert_to_little_endian (SubVI).vi"("string"=w509) -> ("String"=w508:string)  [unwired: 4 in]
            n291 = call "SBG_Ellipse_convert_to_little_endian (SubVI).vi"("string"=w507) -> ("String"=w506:string)  [unwired: 4 in]
            n292 = call "SBG_Ellipse_convert_to_little_endian (SubVI).vi"("string"=w505) -> ("String"=w504:string)  [unwired: 4 in]
            n293 = call "SBG_Ellipse_convert_to_little_endian (SubVI).vi"("string"=w503) -> ("String"=w502:string)  [unwired: 4 in]
            n294 = call "SBG_Ellipse_convert_to_little_endian (SubVI).vi"("string"=w501) -> ("String"=w500:string)  [unwired: 4 in]
            n295 = call "SBG_Ellipse_convert_to_little_endian (SubVI).vi"("string"=w499) -> ("String"=w498:string)  [unwired: 4 in]
            n296 = call "SBG_Ellipse_convert_to_little_endian (SubVI).vi"("string"=w497) -> ("String"=w496:string)  [unwired: 4 in]
            n297 = Type Cast(type=u32 0, x=w482) -> ()  [unwired: 1 out]
            n298 = Type Cast(type=sgl 0.0, x=w484) -> ()  [unwired: 1 out]
            n299 = Type Cast(type=sgl 0.0, x=w508) -> ()  [unwired: 1 out]
            n300 = Type Cast(type=sgl 0.0, x=w506) -> ()  [unwired: 1 out]
            n301 = Type Cast(type=sgl 0.0, x=w504) -> ()  [unwired: 1 out]
            n302 = Type Cast(type=sgl 0.0, x=w502) -> ()  [unwired: 1 out]
            n303 = Type Cast(type=sgl 0.0, x=w500) -> ()  [unwired: 1 out]
            n304 = Type Cast(type=sgl 0.0, x=w498) -> ()  [unwired: 1 out]
            n305 = Type Cast(type=0.0, x=w496) -> ()  [unwired: 1 out]
            n306 = Type Cast(type=u32 0, x=w510) -> ()  [unwired: 1 out]
            n307 = Type Cast(type=0.0, x=w494) -> ()  [unwired: 1 out]
            n308 = Type Cast(type=0.0, x=w492) -> ()  [unwired: 1 out]
            n309 = Type Cast(type=sgl 0.0, x=w490) -> ()  [unwired: 1 out]
            n310 = Type Cast(type=sgl 0.0, x=w488) -> ()  [unwired: 1 out]
            n311 = Type Cast(type=sgl 0.0, x=w486) -> ()  [unwired: 1 out]
          }
        }
      }
      frame "ÿZ\t\u0000.\u0000" {
        w566 = 46 ("x")
        # "SHIP_MOTION 0x09"
        n312 = call "SBG_Ellipse_check_length_n_end (SubVI).vi"("x"=w566, "input String"=w565) -> ("is data ok?"=w564:bool)  [unwired: 7 in, 2 out]
        n313 = case shown="True" w564 {
          tunnel: w565 -> [w567 w633]
          tunnel: [w567 w602] -> w563
          tunnel: w566 -> [_ w616]
          frame False {
          }
          frame True {
            w603 = 6 ("length (len. of substring)")
            # "HEAVE_STATUS"
            # "VEL_Z"
            # "VEL_Y"
            # "VEL_X"
            # "ACC_Z"
            # "ACC_Y"
            # "ACC_X"
            # "HEAVE"
            # "SWAY"
            # "SURGE"
            # "HEAVE PERIOD"
            # "Time Stamp"
            n314 = Replace Substring(2:w616, 3:w603, 5:w633) -> (0:w568:string, 1:w604:string)  [unwired: 1 in]
            n315 = Replace Substring(2:w603, 5:w604) -> (1:w602:string)  [unwired: 2 in, 1 out]
            n316 = String Subset(string=w568, offset (0)=32 ("length (len. of substring)"), length (rest)=4 ("length (len. of substring)")) -> (substring=w583:string)
            n317 = String Subset(string=w568, offset (0)=8 ("length (len. of substring)"), length (rest)=4 ("length (len. of substring)")) -> (substring=w597:string)
            n318 = String Subset(string=w568, offset (0)=4 ("length (len. of substring)"), length (rest)=4 ("length (len. of substring)")) -> (substring=w599:string)
            n319 = String Subset(string=w568, offset (0)=32 ("length (len. of substring)"), length (rest)=4 ("length (len. of substring)")) -> (substring=w584:string)
            n320 = String Subset(string=w568, offset (0)=28 ("length (len. of substring)"), length (rest)=4 ("length (len. of substring)")) -> (substring=w580:string)
            n321 = String Subset(string=w568, offset (0)=12 ("length (len. of substring)"), length (rest)=4 ("length (len. of substring)")) -> (substring=w595:string)
            n322 = String Subset(string=w568, offset (0)=20 ("length (len. of substring)"), length (rest)=4 ("length (len. of substring)")) -> (substring=w591:string)
            n323 = String Subset(string=w568, offset (0)=28 ("length (len. of substring)"), length (rest)=4 ("length (len. of substring)")) -> (substring=w587:string)
            n324 = String Subset(string=w568, offset (0)=24 ("length (len. of substring)"), length (rest)=4 ("length (len. of substring)")) -> (substring=w578:string)
            n325 = String Subset(string=w568, offset (0)=16 ("length (len. of substring)"), length (rest)=4 ("length (len. of substring)")) -> (substring=w593:string)
            n326 = String Subset(string=w568, offset (0)=0 ("length (len. of substring)"), length (rest)=4 ("length (len. of substring)")) -> (substring=w601:string)
            n327 = String Subset(string=w568, offset (0)=24 ("length (len. of substring)"), length (rest)=4 ("length (len. of substring)")) -> (substring=w589:string)
            n328 = call "SBG_Ellipse_convert_to_little_endian (SubVI).vi"("string"=w578) -> ("String"=w579:string)  [unwired: 4 in]
            n329 = call "SBG_Ellipse_convert_to_little_endian (SubVI).vi"("string"=w580) -> ("String"=w581:string)  [unwired: 4 in]
            n330 = call "SBG_Ellipse_convert_to_little_endian (SubVI).vi"("string"=w583) -> ("String"=w582:string)  [unwired: 4 in]
            n331 = call "SBG_Ellipse_convert_to_little_endian (SubVI).vi"("string"=w601) -> ("String"=w600:string)  [unwired: 4 in]
            n332 = call "SBG_Ellipse_convert_to_little_endian (SubVI).vi"("string"=w599) -> ("String"=w598:string)  [unwired: 4 in]
            n333 = call "SBG_Ellipse_convert_to_little_endian (SubVI).vi"("string"=w597) -> ("String"=w596:string)  [unwired: 4 in]
            n334 = call "SBG_Ellipse_convert_to_little_endian (SubVI).vi"("string"=w595) -> ("String"=w594:string)  [unwired: 4 in]
            n335 = call "SBG_Ellipse_convert_to_little_endian (SubVI).vi"("string"=w593) -> ("String"=w592:string)  [unwired: 4 in]
            n336 = call "SBG_Ellipse_convert_to_little_endian (SubVI).vi"("string"=w591) -> ("String"=w590:string)  [unwired: 4 in]
            n337 = call "SBG_Ellipse_convert_to_little_endian (SubVI).vi"("string"=w589) -> ("String"=w588:string)  [unwired: 4 in]
            n338 = call "SBG_Ellipse_convert_to_little_endian (SubVI).vi"("string"=w587) -> ("String"=w586:string)  [unwired: 4 in]
            n339 = call "SBG_Ellipse_convert_to_little_endian (SubVI).vi"("string"=w584) -> ("String"=w585:string)  [unwired: 4 in]
            n340 = Type Cast(type=u16 0, x=w582) -> ()  [unwired: 1 out]
            n341 = Type Cast(type=sgl 0.0, x=w579) -> ()  [unwired: 1 out]
            n342 = Type Cast(type=sgl 0.0, x=w581) -> ()  [unwired: 1 out]
            n343 = Type Cast(type=sgl 0.0, x=w585) -> ()  [unwired: 1 out]
            n344 = Type Cast(type=sgl 0.0, x=w598) -> ()  [unwired: 1 out]
            n345 = Type Cast(type=sgl 0.0, x=w596) -> ()  [unwired: 1 out]
            n346 = Type Cast(type=sgl 0.0, x=w594) -> ()  [unwired: 1 out]
            n347 = Type Cast(type=sgl 0.0, x=w592) -> ()  [unwired: 1 out]
            n348 = Type Cast(type=sgl 0.0, x=w590) -> ()  [unwired: 1 out]
            n349 = Type Cast(type=sgl 0.0, x=w588) -> ()  [unwired: 1 out]
            n350 = Type Cast(type=sgl 0.0, x=w586) -> ()  [unwired: 1 out]
            n351 = Type Cast(type=u32 0, x=w600) -> ()  [unwired: 1 out]
          }
        }
      }
      frame "ÿZ\r\u0000,\u0000" {
        w637 = 44 ("x")
        # "GPS1_Vel 0x0D"
        n352 = call "SBG_Ellipse_check_length_n_end (SubVI).vi"("x"=w637, "input String"=w634) -> ("is data ok?"=w635:bool)  [unwired: 7 in, 2 out]
        n353 = case shown="True" w635 {
          tunnel: w634 -> [w638 w699]
          tunnel: [w638 w661] -> w636
          tunnel: w637 -> [_ w682]
          frame False {
          }
          frame True {
            w662 = 6 ("length (len. of substring)")
            # "course_acc"
            # "course"
            # "vel_acc_d"
            # "vel_acc_e"
            # "vel_acc_n"
            # "Vel_d"
            # "Vel_e"
            # "Vel_n"
            # "GPS_tow"
            # "GPS_Vel_status"
            # "Time Stamp"
            n354 = Replace Substring(2:w682, 3:w662, 5:w699) -> (0:w675:string, 1:w663:string)  [unwired: 1 in]
            n355 = Replace Substring(2:w662, 5:w663) -> (1:w661:string)  [unwired: 2 in, 1 out]
            n356 = String Subset(string=w675, offset (0)=40 ("length (len. of substring)"), length (rest)=4 ("length (len. of substring)")) -> (substring=w640:string)
            n357 = String Subset(string=w675, offset (0)=8 ("length (len. of substring)"), length (rest)=4 ("length (len. of substring)")) -> (substring=w656:string)
            n358 = String Subset(string=w675, offset (0)=36 ("length (len. of substring)"), length (rest)=4 ("length (len. of substring)")) -> (substring=w642:string)
            n359 = String Subset(string=w675, offset (0)=4 ("length (len. of substring)"), length (rest)=4 ("length (len. of substring)")) -> (substring=w658:string)
            n360 = String Subset(string=w675, offset (0)=32 ("length (len. of substring)"), length (rest)=4 ("length (len. of substring)")) -> (substring=w643:string)
            n361 = String Subset(string=w675, offset (0)=12 ("length (len. of substring)"), length (rest)=4 ("length (len. of substring)")) -> (substring=w654:string)
            n362 = String Subset(string=w675, offset (0)=20 ("length (len. of substring)"), length (rest)=4 ("length (len. of substring)")) -> (substring=w650:string)
            n363 = String Subset(string=w675, offset (0)=28 ("length (len. of substring)"), length (rest)=4 ("length (len. of substring)")) -> (substring=w646:string)
            n364 = String Subset(string=w675, offset (0)=16 ("length (len. of substring)"), length (rest)=4 ("length (len. of substring)")) -> (substring=w652:string)
            n365 = String Subset(string=w675, offset (0)=0 ("length (len. of substring)"), length (rest)=4 ("length (len. of substring)")) -> (substring=w660:string)
            n366 = String Subset(string=w675, offset (0)=24 ("length (len. of substring)"), length (rest)=4 ("length (len. of substring)")) -> (substring=w648:string)
            n367 = call "SBG_Ellipse_convert_to_little_endian (SubVI).vi"("string"=w643) -> ("String"=w644:string)  [unwired: 4 in]
            n368 = call "SBG_Ellipse_convert_to_little_endian (SubVI).vi"("string"=w642) -> ("String"=w641:string)  [unwired: 4 in]
            n369 = call "SBG_Ellipse_convert_to_little_endian (SubVI).vi"("string"=w640) -> ("String"=w639:string)  [unwired: 4 in]
            n370 = call "SBG_Ellipse_convert_to_little_endian (SubVI).vi"("string"=w660) -> ("String"=w659:string)  [unwired: 4 in]
            n371 = call "SBG_Ellipse_convert_to_little_endian (SubVI).vi"("string"=w658) -> ("String"=w657:string)  [unwired: 4 in]
            n372 = call "SBG_Ellipse_convert_to_little_endian (SubVI).vi"("string"=w656) -> ("String"=w655:string)  [unwired: 4 in]
            n373 = call "SBG_Ellipse_convert_to_little_endian (SubVI).vi"("string"=w654) -> ("String"=w653:string)  [unwired: 4 in]
            n374 = call "SBG_Ellipse_convert_to_little_endian (SubVI).vi"("string"=w652) -> ("String"=w651:string)  [unwired: 4 in]
            n375 = call "SBG_Ellipse_convert_to_little_endian (SubVI).vi"("string"=w650) -> ("String"=w649:string)  [unwired: 4 in]
            n376 = call "SBG_Ellipse_convert_to_little_endian (SubVI).vi"("string"=w648) -> ("String"=w647:string)  [unwired: 4 in]
            n377 = call "SBG_Ellipse_convert_to_little_endian (SubVI).vi"("string"=w646) -> ("String"=w645:string)  [unwired: 4 in]
            n378 = Type Cast(type=u32 0, x=w659) -> ()  [unwired: 1 out]
            n379 = Type Cast(type=u32 0, x=w657) -> ()  [unwired: 1 out]
            n380 = Type Cast(type=u32 0, x=w655) -> ()  [unwired: 1 out]
            n381 = Type Cast(type=sgl 0.0, x=w645) -> ()  [unwired: 1 out]
            n382 = Type Cast(type=sgl 0.0, x=w644) -> ()  [unwired: 1 out]
            n383 = Type Cast(type=sgl 0.0, x=w641) -> ()  [unwired: 1 out]
            n384 = Type Cast(type=sgl 0.0, x=w639) -> ()  [unwired: 1 out]
            n385 = Type Cast(type=sgl 0.0, x=w653) -> ()  [unwired: 1 out]
            n386 = Type Cast(type=sgl 0.0, x=w651) -> ()  [unwired: 1 out]
            n387 = Type Cast(type=sgl 0.0, x=w649) -> ()  [unwired: 1 out]
            n388 = Type Cast(type=sgl 0.0, x=w647) -> ()  [unwired: 1 out]
          }
        }
      }
      frame "ÿZ\u000e\u00009\u0000" {
        w703 = 57 ("x")
        # "GPS1_Pos 0x0E"
        n389 = call "SBG_Ellipse_check_length_n_end (SubVI).vi"("x"=w703, "input String"=w702) -> ("is data ok?"=w700:bool)  [unwired: 7 in, 2 out]
        n390 = case shown="True" w700 {
          tunnel: w702 -> [w704 w775]
          tunnel: [w704 w733] -> w701
          tunnel: w703 -> [_ w758]
          frame False {
          }
          frame True {
            w732 = 6 ("length (len. of substring)")
            # "diff_age"
            # "base_sation_id"
            # "num_sv_used"
            # "pos_acc_alt"
            # "pos_acc_long"
            # "pos_acc_lat"
            # "undulation"
            # "altitude"
            # "long"
            # "lat"
            # "GPS_tow"
            # "GPS_pos_status"
            # "Time Stamp"
            n391 = Replace Substring(2:w758, 3:w732, 5:w775) -> (0:w747:string, 1:w731:string)  [unwired: 1 in]
            n392 = Replace Substring(2:w732, 5:w731) -> (1:w733:string)  [unwired: 2 in, 1 out]
            n393 = String Subset(string=w747, offset (0)=54 ("length (len. of substring)"), length (rest)=2 ("length (len. of substring)")) -> (substring=w708:string)
            n394 = String Subset(string=w747, offset (0)=56 ("length (len. of substring)"), length (rest)=2 ("length (len. of substring)")) -> (substring=w706:string)
            n395 = String Subset(string=w747, offset (0)=52 ("length (len. of substring)"), length (rest)=1 ("length (len. of substring)")) -> (substring=w709:string)
            n396 = String Subset(string=w747, offset (0)=8 ("length (len. of substring)"), length (rest)=4 ("length (len. of substring)")) -> (substring=w726:string)
            n397 = String Subset(string=w747, offset (0)=48 ("length (len. of substring)"), length (rest)=4 ("length (len. of substring)")) -> (substring=w712:string)
            n398 = String Subset(string=w747, offset (0)=4 ("length (len. of substring)"), length (rest)=4 ("length (len. of substring)")) -> (substring=w728:string)
            n399 = String Subset(string=w747, offset (0)=44 ("length (len. of substring)"), length (rest)=4 ("length (len. of substring)")) -> (substring=w714:string)
            n400 = String Subset(string=w747, offset (0)=12 ("length (len. of substring)"), length (rest)=8 ("length (len. of substring)")) -> (substring=w724:string)
            n401 = String Subset(string=w747, offset (0)=28 ("length (len. of substring)"), length (rest)=8 ("length (len. of substring)")) -> (substring=w720:string)
            n402 = String Subset(string=w747, offset (0)=40 ("length (len. of substring)"), length (rest)=4 ("length (len. of substring)")) -> (substring=w716:string)
            n403 = String Subset(string=w747, offset (0)=20 ("length (len. of substring)"), length (rest)=8 ("length (len. of substring)")) -> (substring=w722:string)
            n404 = String Subset(string=w747, offset (0)=0 ("length (len. of substring)"), length (rest)=4 ("length (len. of substring)")) -> (substring=w730:string)
            n405 = String Subset(string=w747, offset (0)=36 ("length (len. of substring)"), length (rest)=4 ("length (len. of substring)")) -> (substring=w718:string)
            n406 = call "SBG_Ellipse_convert_to_little_endian (SubVI).vi"("string"=w714) -> ("String"=w713:string)  [unwired: 4 in]
            n407 = call "SBG_Ellipse_convert_to_little_endian (SubVI).vi"("string"=w712) -> ("String"=w711:string)  [unwired: 4 in]
            n408 = call "SBG_Ellipse_convert_to_little_endian (SubVI).vi"("string"=w709) -> ("String"=w710:string)  [unwired: 4 in]
            n409 = call "SBG_Ellipse_convert_to_little_endian (SubVI).vi"("string"=w708) -> ("String"=w707:string)  [unwired: 4 in]
            n410 = call "SBG_Ellipse_convert_to_little_endian (SubVI).vi"("string"=w706) -> ("String"=w705:string)  [unwired: 4 in]
            n411 = call "SBG_Ellipse_convert_to_little_endian (SubVI).vi"("string"=w730) -> ("String"=w729:string)  [unwired: 4 in]
            n412 = call "SBG_Ellipse_convert_to_little_endian (SubVI).vi"("string"=w728) -> ("String"=w727:string)  [unwired: 4 in]
            n413 = call "SBG_Ellipse_convert_to_little_endian (SubVI).vi"("string"=w726) -> ("String"=w725:string)  [unwired: 4 in]
            n414 = call "SBG_Ellipse_convert_to_little_endian (SubVI).vi"("string"=w724) -> ("String"=w723:string)  [unwired: 4 in]
            n415 = call "SBG_Ellipse_convert_to_little_endian (SubVI).vi"("string"=w722) -> ("String"=w721:string)  [unwired: 4 in]
            n416 = call "SBG_Ellipse_convert_to_little_endian (SubVI).vi"("string"=w720) -> ("String"=w719:string)  [unwired: 4 in]
            n417 = call "SBG_Ellipse_convert_to_little_endian (SubVI).vi"("string"=w718) -> ("String"=w717:string)  [unwired: 4 in]
            n418 = call "SBG_Ellipse_convert_to_little_endian (SubVI).vi"("string"=w716) -> ("String"=w715:string)  [unwired: 4 in]
            n419 = Type Cast(type=u32 0, x=w729) -> ()  [unwired: 1 out]
            n420 = Type Cast(type=u32 0, x=w727) -> ()  [unwired: 1 out]
            n421 = Type Cast(type=u32 0, x=w725) -> ()  [unwired: 1 out]
            n422 = Type Cast(type=0.0, x=w723) -> ()  [unwired: 1 out]
            n423 = Type Cast(type=0.0, x=w721) -> ()  [unwired: 1 out]
            n424 = Type Cast(type=0.0, x=w719) -> ()  [unwired: 1 out]
            n425 = Type Cast(type=sgl 0.0, x=w717) -> ()  [unwired: 1 out]
            n426 = Type Cast(type=sgl 0.0, x=w715) -> ()  [unwired: 1 out]
            n427 = Type Cast(type=sgl 0.0, x=w713) -> ()  [unwired: 1 out]
            n428 = Type Cast(type=sgl 0.0, x=w711) -> ()  [unwired: 1 out]
            n429 = Type Cast(type=u8 0, x=w710) -> ()  [unwired: 1 out]
            n430 = Type Cast(type=u16 0, x=w707) -> ()  [unwired: 1 out]
            n431 = Type Cast(type=u16 0, x=w705) -> ()  [unwired: 1 out]
          }
        }
      }
      frame "ÿZ\u000f\u0000\u001a\u0000" {
        w779 = 26 ("x")
        # "GPS1_HDT 0x0F"
        n432 = call "SBG_Ellipse_check_length_n_end (SubVI).vi"("x"=w779, "input String"=w778) -> ("is data ok?"=w776:bool)  [unwired: 7 in, 2 out]
        n433 = case shown="True" w776 {
          tunnel: w778 -> [w780 w821]
          tunnel: [w780 w797] -> w777
          tunnel: w779 -> [_ w806]
          frame False {
          }
          frame True {
            w795 = 6 ("length (len. of substring)")
            # "GPS PITCH ACC"
            # "GPS PITCH"
            # "GPS HEADING ACC"
            # "GPS TRUE HEADING"
            # "GPS_tow"
            # "GPS HDT STATUS"
            # "Time Stamp"
            n434 = Replace Substring(2:w806, 3:w795, 5:w821) -> (0:w805:string, 1:w796:string)  [unwired: 1 in]
            n435 = Replace Substring(2:w795, 5:w796) -> (1:w797:string)  [unwired: 2 in, 1 out]
            n436 = String Subset(string=w805, offset (0)=6 ("length (len. of substring)"), length (rest)=4 ("length (len. of substring)")) -> (substring=w782:string)
            n437 = String Subset(string=w805, offset (0)=4 ("length (len. of substring)"), length (rest)=2 ("length (len. of substring)")) -> (substring=w792:string)
            n438 = String Subset(string=w805, offset (0)=10 ("length (len. of substring)"), length (rest)=4 ("length (len. of substring)")) -> (substring=w784:string)
            n439 = String Subset(string=w805, offset (0)=18 ("length (len. of substring)"), length (rest)=4 ("length (len. of substring)")) -> (substring=w788:string)
            n440 = String Subset(string=w805, offset (0)=14 ("length (len. of substring)"), length (rest)=4 ("length (len. of substring)")) -> (substring=w786:string)
            n441 = String Subset(string=w805, offset (0)=0 ("length (len. of substring)"), length (rest)=4 ("length (len. of substring)")) -> (substring=w794:string)
            n442 = String Subset(string=w805, offset (0)=22 ("length (len. of substring)"), length (rest)=4 ("length (len. of substring)")) -> (substring=w790:string)
            n443 = call "SBG_Ellipse_convert_to_little_endian (SubVI).vi"("string"=w794) -> ("String"=w793:string)  [unwired: 4 in]
            n444 = call "SBG_Ellipse_convert_to_little_endian (SubVI).vi"("string"=w792) -> ("String"=w791:string)  [unwired: 4 in]
            n445 = call "SBG_Ellipse_convert_to_little_endian (SubVI).vi"("string"=w782) -> ("String"=w781:string)  [unwired: 4 in]
            n446 = call "SBG_Ellipse_convert_to_little_endian (SubVI).vi"("string"=w784) -> ("String"=w783:string)  [unwired: 4 in]
            n447 = call "SBG_Ellipse_convert_to_little_endian (SubVI).vi"("string"=w786) -> ("String"=w785:string)  [unwired: 4 in]
            n448 = call "SBG_Ellipse_convert_to_little_endian (SubVI).vi"("string"=w788) -> ("String"=w787:string)  [unwired: 4 in]
            n449 = call "SBG_Ellipse_convert_to_little_endian (SubVI).vi"("string"=w790) -> ("String"=w789:string)  [unwired: 4 in]
            n450 = Type Cast(type=u32 0, x=w793) -> ()  [unwired: 1 out]
            n451 = Type Cast(type=u16 0, x=w791) -> ()  [unwired: 1 out]
            n452 = Type Cast(type=u32 0, x=w781) -> ()  [unwired: 1 out]
            n453 = Type Cast(type=sgl 0.0, x=w783) -> ()  [unwired: 1 out]
            n454 = Type Cast(type=sgl 0.0, x=w785) -> ()  [unwired: 1 out]
            n455 = Type Cast(type=sgl 0.0, x=w787) -> ()  [unwired: 1 out]
            n456 = Type Cast(type=sgl 0.0, x=w789) -> ()  [unwired: 1 out]
          }
        }
      }
      frame "ÿZ\u0013\u0000\n\u0000" {
        w825 = 10 ("x")
        # "ODO_VEL 0x13"
        n457 = call "SBG_Ellipse_check_length_n_end (SubVI).vi"("x"=w825, "input String"=w824) -> ("is data ok?"=w822:bool)  [unwired: 7 in, 2 out]
        n458 = case shown="True" w822 {
          tunnel: w824 -> [w826 w848]
          tunnel: [w826 w834] -> w823
          tunnel: w825 -> [_ w841]
          frame False {
          }
          frame True {
            w835 = 6 ("length (len. of substring)")
            # "ODO_VEL"
            # "ODO_STATUS"
            # "Time Stamp"
            n459 = Replace Substring(2:w841, 3:w835, 5:w848) -> (0:w840:string, 1:w836:string)  [unwired: 1 in]
            n460 = Replace Substring(2:w835, 5:w836) -> (1:w834:string)  [unwired: 2 in, 1 out]
            n461 = String Subset(string=w840, offset (0)=6 ("length (len. of substring)"), length (rest)=4 ("length (len. of substring)")) -> (substring=w829:string)
            n462 = String Subset(string=w840, offset (0)=4 ("length (len. of substring)"), length (rest)=2 ("length (len. of substring)")) -> (substring=w831:string)
            n463 = String Subset(string=w840, offset (0)=0 ("length (len. of substring)"), length (rest)=4 ("length (len. of substring)")) -> (substring=w833:string)
            n464 = call "SBG_Ellipse_convert_to_little_endian (SubVI).vi"("string"=w833) -> ("String"=w832:string)  [unwired: 4 in]
            n465 = call "SBG_Ellipse_convert_to_little_endian (SubVI).vi"("string"=w831) -> ("String"=w830:string)  [unwired: 4 in]
            n466 = call "SBG_Ellipse_convert_to_little_endian (SubVI).vi"("string"=w829) -> ("String"=w828:string)  [unwired: 4 in]
            n467 = Type Cast(type=u16 0, x=w830) -> ()  [unwired: 1 out]
            n468 = Type Cast(type=sgl 0.0, x=w828) -> (*(type *) &x=w827:sgl)
            n469 = Type Cast(type=u32 0, x=w832) -> ()  [unwired: 1 out]
            n470 = To Double Precision Float(number=w827) -> ()  [unwired: 1 out]
          }
        }
      }
      frame "ÿZ\u0018\u0000\u000e\u0000" {
        w852 = 14 ("x")
        # "EVENT_A 0x18"
        # "EVENT_A 0x18"
        n471 = call "SBG_Ellipse_check_length_n_end (SubVI).vi"("x"=w852, "input String"=w851) -> ("is data ok?"=w849:bool)  [unwired: 7 in, 2 out]
        n472 = case shown="True" w849 {
          tunnel: w851 -> [w853 w889]
          tunnel: [w853 w867] -> w850
          tunnel: w852 -> [_ w876]
          frame False {
          }
          frame True {
            w866 = 6 ("length (len. of substring)")
            # "TIME OFFSET_3"
            # "TIME OFFSET_2"
            # "TIME OFFSET_1"
            # "TIME OFFSET_0"
            # "EVENT STATUS"
            # "Time Stamp"
            n473 = Replace Substring(2:w876, 3:w866, 5:w889) -> (0:w875:string, 1:w868:string)  [unwired: 1 in]
            n474 = Replace Substring(2:w866, 5:w868) -> (1:w867:string)  [unwired: 2 in, 1 out]
            n475 = String Subset(string=w875, offset (0)=6 ("length (len. of substring)"), length (rest)=2 ("length (len. of substring)")) -> (substring=w861:string)
            n476 = String Subset(string=w875, offset (0)=4 ("length (len. of substring)"), length (rest)=2 ("length (len. of substring)")) -> (substring=w863:string)
            n477 = String Subset(string=w875, offset (0)=8 ("length (len. of substring)"), length (rest)=2 ("length (len. of substring)")) -> (substring=w859:string)
            n478 = String Subset(string=w875, offset (0)=12 ("length (len. of substring)"), length (rest)=2 ("length (len. of substring)")) -> (substring=w855:string)
            n479 = String Subset(string=w875, offset (0)=10 ("length (len. of substring)"), length (rest)=2 ("length (len. of substring)")) -> (substring=w857:string)
            n480 = String Subset(string=w875, offset (0)=0 ("length (len. of substring)"), length (rest)=4 ("length (len. of substring)")) -> (substring=w865:string)
            n481 = call "SBG_Ellipse_convert_to_little_endian (SubVI).vi"("string"=w865) -> ("String"=w864:string)  [unwired: 4 in]
            n482 = call "SBG_Ellipse_convert_to_little_endian (SubVI).vi"("string"=w863) -> ("String"=w862:string)  [unwired: 4 in]
            n483 = call "SBG_Ellipse_convert_to_little_endian (SubVI).vi"("string"=w861) -> ("String"=w860:string)  [unwired: 4 in]
            n484 = call "SBG_Ellipse_convert_to_little_endian (SubVI).vi"("string"=w859) -> ("String"=w858:string)  [unwired: 4 in]
            n485 = call "SBG_Ellipse_convert_to_little_endian (SubVI).vi"("string"=w857) -> ("String"=w856:string)  [unwired: 4 in]
            n486 = call "SBG_Ellipse_convert_to_little_endian (SubVI).vi"("string"=w855) -> ("String"=w854:string)  [unwired: 4 in]
            n487 = Type Cast(type=u32 0, x=w864) -> ()  [unwired: 1 out]
            n488 = Type Cast(type=u16 0, x=w862) -> ()  [unwired: 1 out]
            n489 = Type Cast(type=u16 0, x=w860) -> ()  [unwired: 1 out]
            n490 = Type Cast(type=u16 0, x=w858) -> ()  [unwired: 1 out]
            n491 = Type Cast(type=u16 0, x=w856) -> ()  [unwired: 1 out]
            n492 = Type Cast(type=u16 0, x=w854) -> ()  [unwired: 1 out]
          }
        }
      }
      frame "ÿZ$\u0000\u000e\u0000" {
        w893 = 14 ("x")
        # "PRESSURE 0x24"
        n493 = call "SBG_Ellipse_check_length_n_end (SubVI).vi"("x"=w893, "input String"=w892) -> ("is data ok?"=w890:bool)  [unwired: 7 in, 2 out]
        n494 = case shown="True" w890 {
          tunnel: w892 -> [w894 w924]
          tunnel: [w894 w907] -> w891
          tunnel: w893 -> [_ w915]
          frame False {
          }
          frame True {
            w908 = 6 ("length (len. of substring)")
            # "Altitude"
            # "Pressure"
            # "Pressure_status"
            # "Time Stamp"
            n495 = Replace Substring(2:w915, 3:w908, 5:w924) -> (0:w914:string, 1:w909:string)  [unwired: 1 in]
            n496 = Replace Substring(2:w908, 5:w909) -> (1:w907:string)  [unwired: 2 in, 1 out]
            n497 = String Subset(string=w914, offset (0)=6 ("length (len. of substring)"), length (rest)=4 ("length (len. of substring)")) -> (substring=w902:string)
            n498 = String Subset(string=w914, offset (0)=4 ("length (len. of substring)"), length (rest)=2 ("length (len. of substring)")) -> (substring=w904:string)
            n499 = String Subset(string=w914, offset (0)=10 ("length (len. of substring)"), length (rest)=4 ("length (len. of substring)")) -> (substring=w900:string)
            n500 = String Subset(string=w914, offset (0)=0 ("length (len. of substring)"), length (rest)=4 ("length (len. of substring)")) -> (substring=w906:string)
            n501 = call "SBG_Ellipse_convert_to_little_endian (SubVI).vi"("string"=w906) -> ("String"=w905:string)  [unwired: 4 in]
            n502 = call "SBG_Ellipse_convert_to_little_endian (SubVI).vi"("string"=w904) -> ("String"=w903:string)  [unwired: 4 in]
            n503 = call "SBG_Ellipse_convert_to_little_endian (SubVI).vi"("string"=w902) -> ("String"=w901:string)  [unwired: 4 in]
            n504 = call "SBG_Ellipse_convert_to_little_endian (SubVI).vi"("string"=w900) -> ("String"=w899:string)  [unwired: 4 in]
            n505 = Type Cast(type=u16 0, x=w903) -> ()  [unwired: 1 out]
            n506 = Type Cast(type=sgl 0.0, x=w901) -> (*(type *) &x=w898:sgl)
            n507 = Type Cast(type=sgl 0.0, x=w899) -> ()  [unwired: 1 out]
            n508 = Type Cast(type=u32 0, x=w905) -> ()  [unwired: 1 out]
            n509 = To Double Precision Float(number=w898) -> (double precision float=w895:dbl)
            n510 = shared-variable ".\\MasterLocalVariables.lvlib\\IMUData"() -> (w896:T2)  [unwired: 1 in, 1 out]
            n511 = Bundle By Name(cluster=w896, "Pressure (psia)"=w895) -> (w897:T2)
            n512 = shared-variable ".\\MasterLocalVariables.lvlib\\IMUData"(w897) -> ()  [unwired: 1 in, 1 out]
          }
        }
      }
    }
    n513 = call "SBG_Ellipse_starting_debug (SubVI).vi"("boolean from check"=w6, "result string in"=w9) -> ("result string out"=w14:string)  [unwired: 9 in]
    n514 = String Length(string=w14) -> (length=w17:i32)
    "buffer length" <- w17
    n515 = Greater Or Equal?(x=w17, y=10000) -> (x >= y?=w15:bool)
    n516 = Select(t="", s=w15, f=w14) -> (s? t:f=w12:string)
    n517 = feedback-in #1(w12) -> ()
    n518 = shared-variable ".\\MasterLocalVariables.lvlib\\GlobalStop"() -> (w10:bool)  [unwired: 1 in, 1 out]
  }
  "error out" <- w3
